vi "TestM1M3SALEvents.vi"() -> ()   [LabVIEW 2016]
uses:
  Communicator/M1M3SAL/M1M3SAL.lvclass
  Communicator/DataTypes/M1M3SALSettings.ctl
  UserEvents/UserEvents.lvclass
  DataTypes/General/ShutdownEvent.ctl
  Communicator/M1M3SAL/M1M3SAL.lvclass/M1M3SAL.ctl
  UserEvents/UserEvents.lvclass/UserEvents.ctl
  DataTypes/Topics/EventActuatorBroadcastCounter.ctl
  DataTypes/Topics/Parts/Timestamp.ctl
  DataTypes/Topics/EventActuatorTestStatus.ctl
  DataTypes/Topics/EventAirStatus.ctl
  DataTypes/Topics/EventAppliedSettingsMatchStart.ctl
  DataTypes/Topics/EventCellChecks.ctl
  DataTypes/Topics/EventDetailedState.ctl
  DataTypes/Topics/Parts/DetailedStates.ctl
  DataTypes/Topics/EventElevationAngleChecks.ctl
  DataTypes/Topics/EventForceActuatorSafetyChecks.ctl
  DataTypes/Topics/EventErrorCode.ctl
  DataTypes/Topics/EventForceActuatorInfo.ctl
  DataTypes/Topics/EventHardpointActuatorInfo.ctl
  DataTypes/Topics/EventForceActuatorTest.ctl
  DataTypes/Topics/Parts/TestStatus.ctl
  DataTypes/Topics/EventHardpointActuatorBreakaway.ctl
  DataTypes/Topics/EventHardpointActuatorChase.ctl
  DataTypes/Topics/EventILCCommunication.ctl
  DataTypes/Topics/EventLowerMirrorComplete.ctl
  DataTypes/Topics/EventRaiseMirrorComplete.ctl
  DataTypes/Topics/EventServoLoops.ctl
  DataTypes/Topics/EventSettingsApplied.ctl
  DataTypes/Topics/EventSettingVersions.ctl
  DataTypes/Topics/EventStartupChecks.ctl
  DataTypes/Topics/EventStatusChecks.ctl
  DataTypes/Topics/EventSummaryState.ctl
  DataTypes/Topics/Parts/SummaryStates.ctl
  Communicator/M1M3SupportCommunicator.lvlib
  DataTypes/Topics/M1M3SupportTopics.lvlib
  DataTypes/General/M1M3SupportGeneral.lvlib
panel:
  out "SummaryState":bool
  out "StatusChecks":bool
  out "StartupChecks":bool
  out "SettingVersions":bool
  out "SettingsApplied":bool
  out "ServoLoops":bool
  out "RaiseMirrorComplete":bool
  out "LowerMirrorComplete":bool
  out "ILCCommunication":bool
  out "HardpointActuatorInfo":bool
  out "HardpointActuatorChase":bool
  out "HardpointActuatorBreakaway":bool
  out "ForceActuatorTest":bool
  in  "SummaryStateGo":bool
  in  "StatusChecksGo":bool
  in  "StartupChecksGo":bool
  in  "SettingVersionsGo":bool
  in  "SettingsAppliedGo":bool
  in  "ServoLoopsGo":bool
  in  "RaiseMirrorCompleteGo":bool
  in  "LowerMirrorCompleteGo":bool
  in  "ILCCommunicationGo":bool
  in  "HardpointActuatorInfoGo":bool
  in  "HardpointActuatorChaseGo":bool
  in  "HardpointActuatorBreakawayGo":bool
  in  "ForceActuatorTestGo":bool
  out "ForceActuatorSafetyChecks":bool
  in  "ForceActuatorSafetyChecksGo":bool
  out "ForceActuatorInfo":bool
  out "ErrorCode":bool
  out "ElevationAngleChecks":bool
  in  "ForceActuatorInfoGo":bool
  in  "ErrorCodeGo":bool
  in  "ElevationAngleChecksGo":bool
  out "DetailedState":bool
  out "CellChecks":bool
  out "AppliedSettingsMatchStart":bool
  out "AirStatus":bool
  in  "DetailedStateGo":bool
  in  "CellChecksGo":bool
  in  "AppliedSettingsMatchStartGo":bool
  in  "AirStatusGo":bool
  in  "ActuatorTestStatusGo":bool
  out "ActuatorTestStatus":bool
  out "Ready?":bool
  in  "ActuatorBroadcastCounterGo":bool
  out "ActuatorBroadcastCounter":bool
  in  "Stop":bool
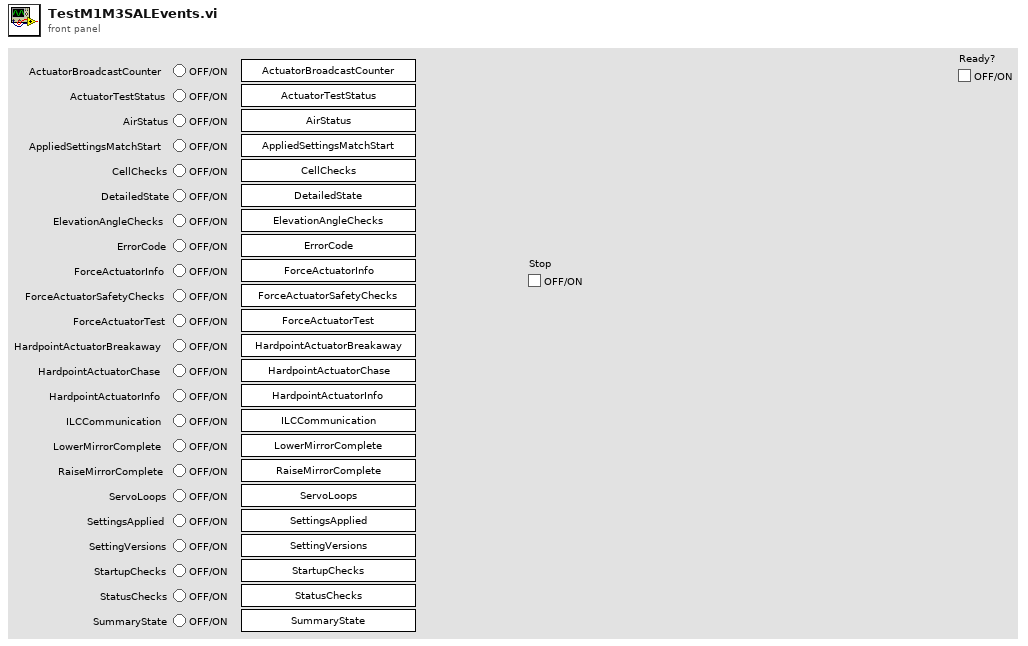
[diagram p1: front panel]
types:
  T1 = typedef "M1M3SupportGeneral.lvlib/ShutdownEvent.ctl" = cluster{"Shutdown":bool}
  T2 = typedef "M1M3SupportCommunicator.lvlib/M1M3SALSettings.ctl" = cluster{"IPAddress":string, "Port":u16, "StartupScript":string}
  T3 = typedef "M1M3SupportTopics.lvlib/Timestamp.ctl" = dbl
  T4 = typedef "M1M3SupportTopics.lvlib/DetailedStates.ctl" = enum16{"OfflineState", "InitialState", "StandbyState", "DisabledState", "ParkedState", "FaultState", "ParkedMaintenanceState", "ActiveMaintenanceState"}
  T5 = typedef "M1M3SupportTopics.lvlib/TestStatus.ctl" = enum16{"NotRun", "Pass", "Fail"}
  T6 = typedef "M1M3SupportTopics.lvlib/SummaryStates.ctl" = enum16{"OfflineState", "StandbyState", "DisabledState", "EnabledState", "FaultState"}
  T7 = typedef "M1M3SupportTypes.lvlib/Timestamp.ctl" = dbl
  T8 = typedef "M1M3SupportTypes.lvlib/SummaryStates.ctl" = enum16{"OfflineState", "StandbyState", "DisabledState", "EnabledState", "FaultState"}
  T9 = typedef "M1M3SupportTopics.lvlib/EventActuatorBroadcastCounter.ctl" = cluster{"Timestamp":T3, "ActuatorId":i32, "CounterOk":bool}
  T10 = typedef "M1M3SupportTopics.lvlib/EventActuatorTestStatus.ctl" = cluster{"Timestamp":T3, "AllTestsRan":bool}
  T11 = typedef "M1M3SupportTopics.lvlib/EventAirStatus.ctl" = cluster{"Timestamp":T3, "AirCommandedOn":bool, "AirOn":bool, "AirPressureOk":bool, "HardpointAirPressureOk":bool}
  T12 = typedef "M1M3SupportTopics.lvlib/EventAppliedSettingsMatchStart.ctl" = cluster{"Timestamp":T3, "AppliedSettingsMatchStart":bool}
  T13 = typedef "M1M3SupportTopics.lvlib/EventCellChecks.ctl" = cluster{"Timestamp":T3, "MirrorDoorClosed":bool}
  T14 = typedef "M1M3SupportTopics.lvlib/EventDetailedState.ctl" = cluster{"Timestamp":T3, "DetailedStates":T4}
  T15 = typedef "M1M3SupportTopics.lvlib/EventElevationAngleChecks.ctl" = cluster{"Timestamp":T3, "MatchesTMA":bool, "MatchesInclinometer":bool, "MatchesMeasured":bool}
  T16 = typedef "M1M3SupportTopics.lvlib/EventForceActuatorSafetyChecks.ctl" = cluster{"Timestamp":T3, "AllInSafetyLimit":bool, "SafetyLimitOk":bool[], "MirrorWeightOk":bool, "XMomentOk":bool, "YMomentOk":bool, "AllNeighborsOk":bool, "NeighborsOk":bool[], "MagnitudeOk":bool, "AllGlobalBendingOk":bool, "GlobalBendingOk":bool[], "FollowingErrorOk":bool, "AxialFollowingErrorOk":bool[], "LateralFollowingErrorOk":bool[], "AOSNetForceOk":bool, "AllElevationForcesOk":bool, "ElevationForcesOk":bool[], "AllAzimuthForcesOk":bool, "AzimuthForcesOk":bool[], "AllThermalForcesOk":bool, "ThermalForcesOk":bool[], "AllAOSForcesOk":bool, "AOSForcesOk":bool[]}
  T17 = typedef "M1M3SupportTopics.lvlib/EventErrorCode.ctl" = cluster{"Timestamp":T3, "ErrorCode":i32}
  T18 = typedef "M1M3SupportTopics.lvlib/EventForceActuatorInfo.ctl" = cluster{"Timestamp":T3, "ReferenceId":i32[], "XPosition":sgl[], "YPosition":sgl[], "ZPosition":sgl[], "ILCUniqueId":i64[], "ILCApplicationType":u8[], "NetworkNodeType":u8[], "ILCSelectedOptions":u8[], "NetworkNodeOptions":u8[], "MajorRevision":u8[], "MinorRevision":u8[], "ADCScanRate":u8[], "MainADCCalibrationK1":sgl[], "MainADCCalibrationK2":sgl[], "MainADCCalibrationK3":sgl[], "MainADCCalibrationK4":sgl[], "MainAxialLoadCellOffset":sgl[], "MainLateralLoadCellOffset":sgl[], "MainAxialLoadCellSensitivity":sgl[], "MainLateralLoadCellSensitivity":sgl[], "BackupADCCalibrationK1":sgl[], "BackupADCCalibrationK2":sgl[], "BackupADCCalibrationK3":sgl[], "BackupADCCalibrationK4":sgl[], "BackupAxialLoadCellOffset":sgl[], "BackupLateralLoadCellOffset":sgl[], "BackupAxialLoadCellSensitivity":sgl[], "BackupLateralLoadCellSensitivity":sgl[], "DCAAxialGain":sgl[], "DCALateralGain":sgl[], "DCAUniqueId":i64[], "DCAFirmwareType":u8[], "DCAMajorRevision":u8[], "DCAMinorRevision":u8[], "MainCalibrationError":bool[], "BackupCalibrationError":bool[], "DCAFirmwareUpdate":bool[], "UniqueIdCRCError":bool[], "ApplicationTypeMismatch":bool[], "ApplicationMissing":bool[], "ApplicationCRCMismatch":bool[], "OneWireMissing":bool[], "OneWire1Mismatch":bool[], "OneWire2Mismatch":bool[], "DCAUniqueIdCRCError":bool[], "DCAMainCalibrationError":bool[], "DCABackupCalibrationError":bool[], "DCAApplicationMissing":bool[], "DCAApplicationCRCMismatch":bool[], "DCABootloaderActive":bool[]}
  T19 = typedef "M1M3SupportTopics.lvlib/EventHardpointActuatorInfo.ctl" = cluster{"Timestamp":T3, "ReferenceId":i32[], "ReferencePosition":i32[], "XPosition":sgl[], "YPosition":sgl[], "ZPosition":sgl[], "ILCUniqueId":i64[], "ILCApplicationType":u8[], "NetworkNodeType":u8[], "ILCSelectedOptions":u8[], "NetworkNodeOptions":u8[], "MajorRevision":u8[], "MinorRevision":u8[], "ADCScanRate":u8[], "MainADCCalibrationK1":sgl[], "MainADCCalibrationK2":sgl[], "MainADCCalibrationK3":sgl[], "MainADCCalibrationK4":sgl[], "MainLoadCellOffset":sgl[], "MainLoadCellSensitivity":sgl[], "BackupADCCalibrationK1":sgl[], "BackupADCCalibrationK2":sgl[], "BackupADCCalibrationK3":sgl[], "BackupADCCalibrationK4":sgl[], "BackupLoadCellOffset":sgl[], "BackupLoadCellSensitivity":sgl[], "MainCalibrationError":bool[], "BackupCalibrationError":bool[], "UniqueIdCRCError":bool[], "ApplicationTypeMismatch":bool[], "ApplicationMissing":bool[], "ApplicationCRCMismatch":bool[], "OneWireMissing":bool[], "OneWire1Mismatch":bool[], "OneWire2Mismatch":bool[]}
  T20 = typedef "M1M3SupportTopics.lvlib/EventForceActuatorTest.ctl" = cluster{"Timestamp":T3, "ActuatorId":i32, "TestStatus":T5}
  T21 = typedef "M1M3SupportTopics.lvlib/EventHardpointActuatorBreakaway.ctl" = cluster{"Timestamp":T3, "ActuatorId":i32, "ForceOk":bool}
  T22 = typedef "M1M3SupportTopics.lvlib/EventHardpointActuatorChase.ctl" = cluster{"Timestamp":T3, "ActuatorId":i32, "Chasing":bool}
  T23 = typedef "M1M3SupportTopics.lvlib/EventILCCommunication.ctl" = cluster{"Timestamp":T3, "ActuatorId":i32, "CommunicationOK":bool}
  T24 = typedef "M1M3SupportTopics.lvlib/EventLowerMirrorComplete.ctl" = cluster{"Timestamp":T3, "Successful":bool}
  T25 = typedef "M1M3SupportTopics.lvlib/EventRaiseMirrorComplete.ctl" = cluster{"Timestamp":T3, "Successful":bool}
  T26 = typedef "M1M3SupportTopics.lvlib/EventServoLoops.ctl" = cluster{"Timestamp":T3, "HardpointChase":bool, "HardpointOffloading":bool, "OuterLoopTimeOk":bool}
  T27 = typedef "M1M3SupportTopics.lvlib/EventSettingsApplied.ctl" = cluster{"Timestamp":T3, "Settings":string}
  T28 = typedef "M1M3SupportTopics.lvlib/EventSettingVersions.ctl" = cluster{"Timestamp":T3, "RecommendedSettingsVersion":string}
  T29 = typedef "M1M3SupportTopics.lvlib/EventStartupChecks.ctl" = cluster{"Timestamp":T3, "ILCVersionsOk":bool, "DCAVersionsOk":bool, "ILCFirmwareOk":bool, "DCAFirmwareOk":bool, "ILCStatusOk":bool, "DCAStatusOk":bool}
  T30 = typedef "M1M3SupportTopics.lvlib/EventStatusChecks.ctl" = cluster{"Timestamp":T3, "ILCResetOk":bool, "DCAResetOk":bool, "ILCPowerOk":bool, "DCAPowerOk":bool}
  T31 = typedef "M1M3SupportTopics.lvlib/EventSummaryState.ctl" = cluster{"Timestamp":T3, "SummaryStates":T6}
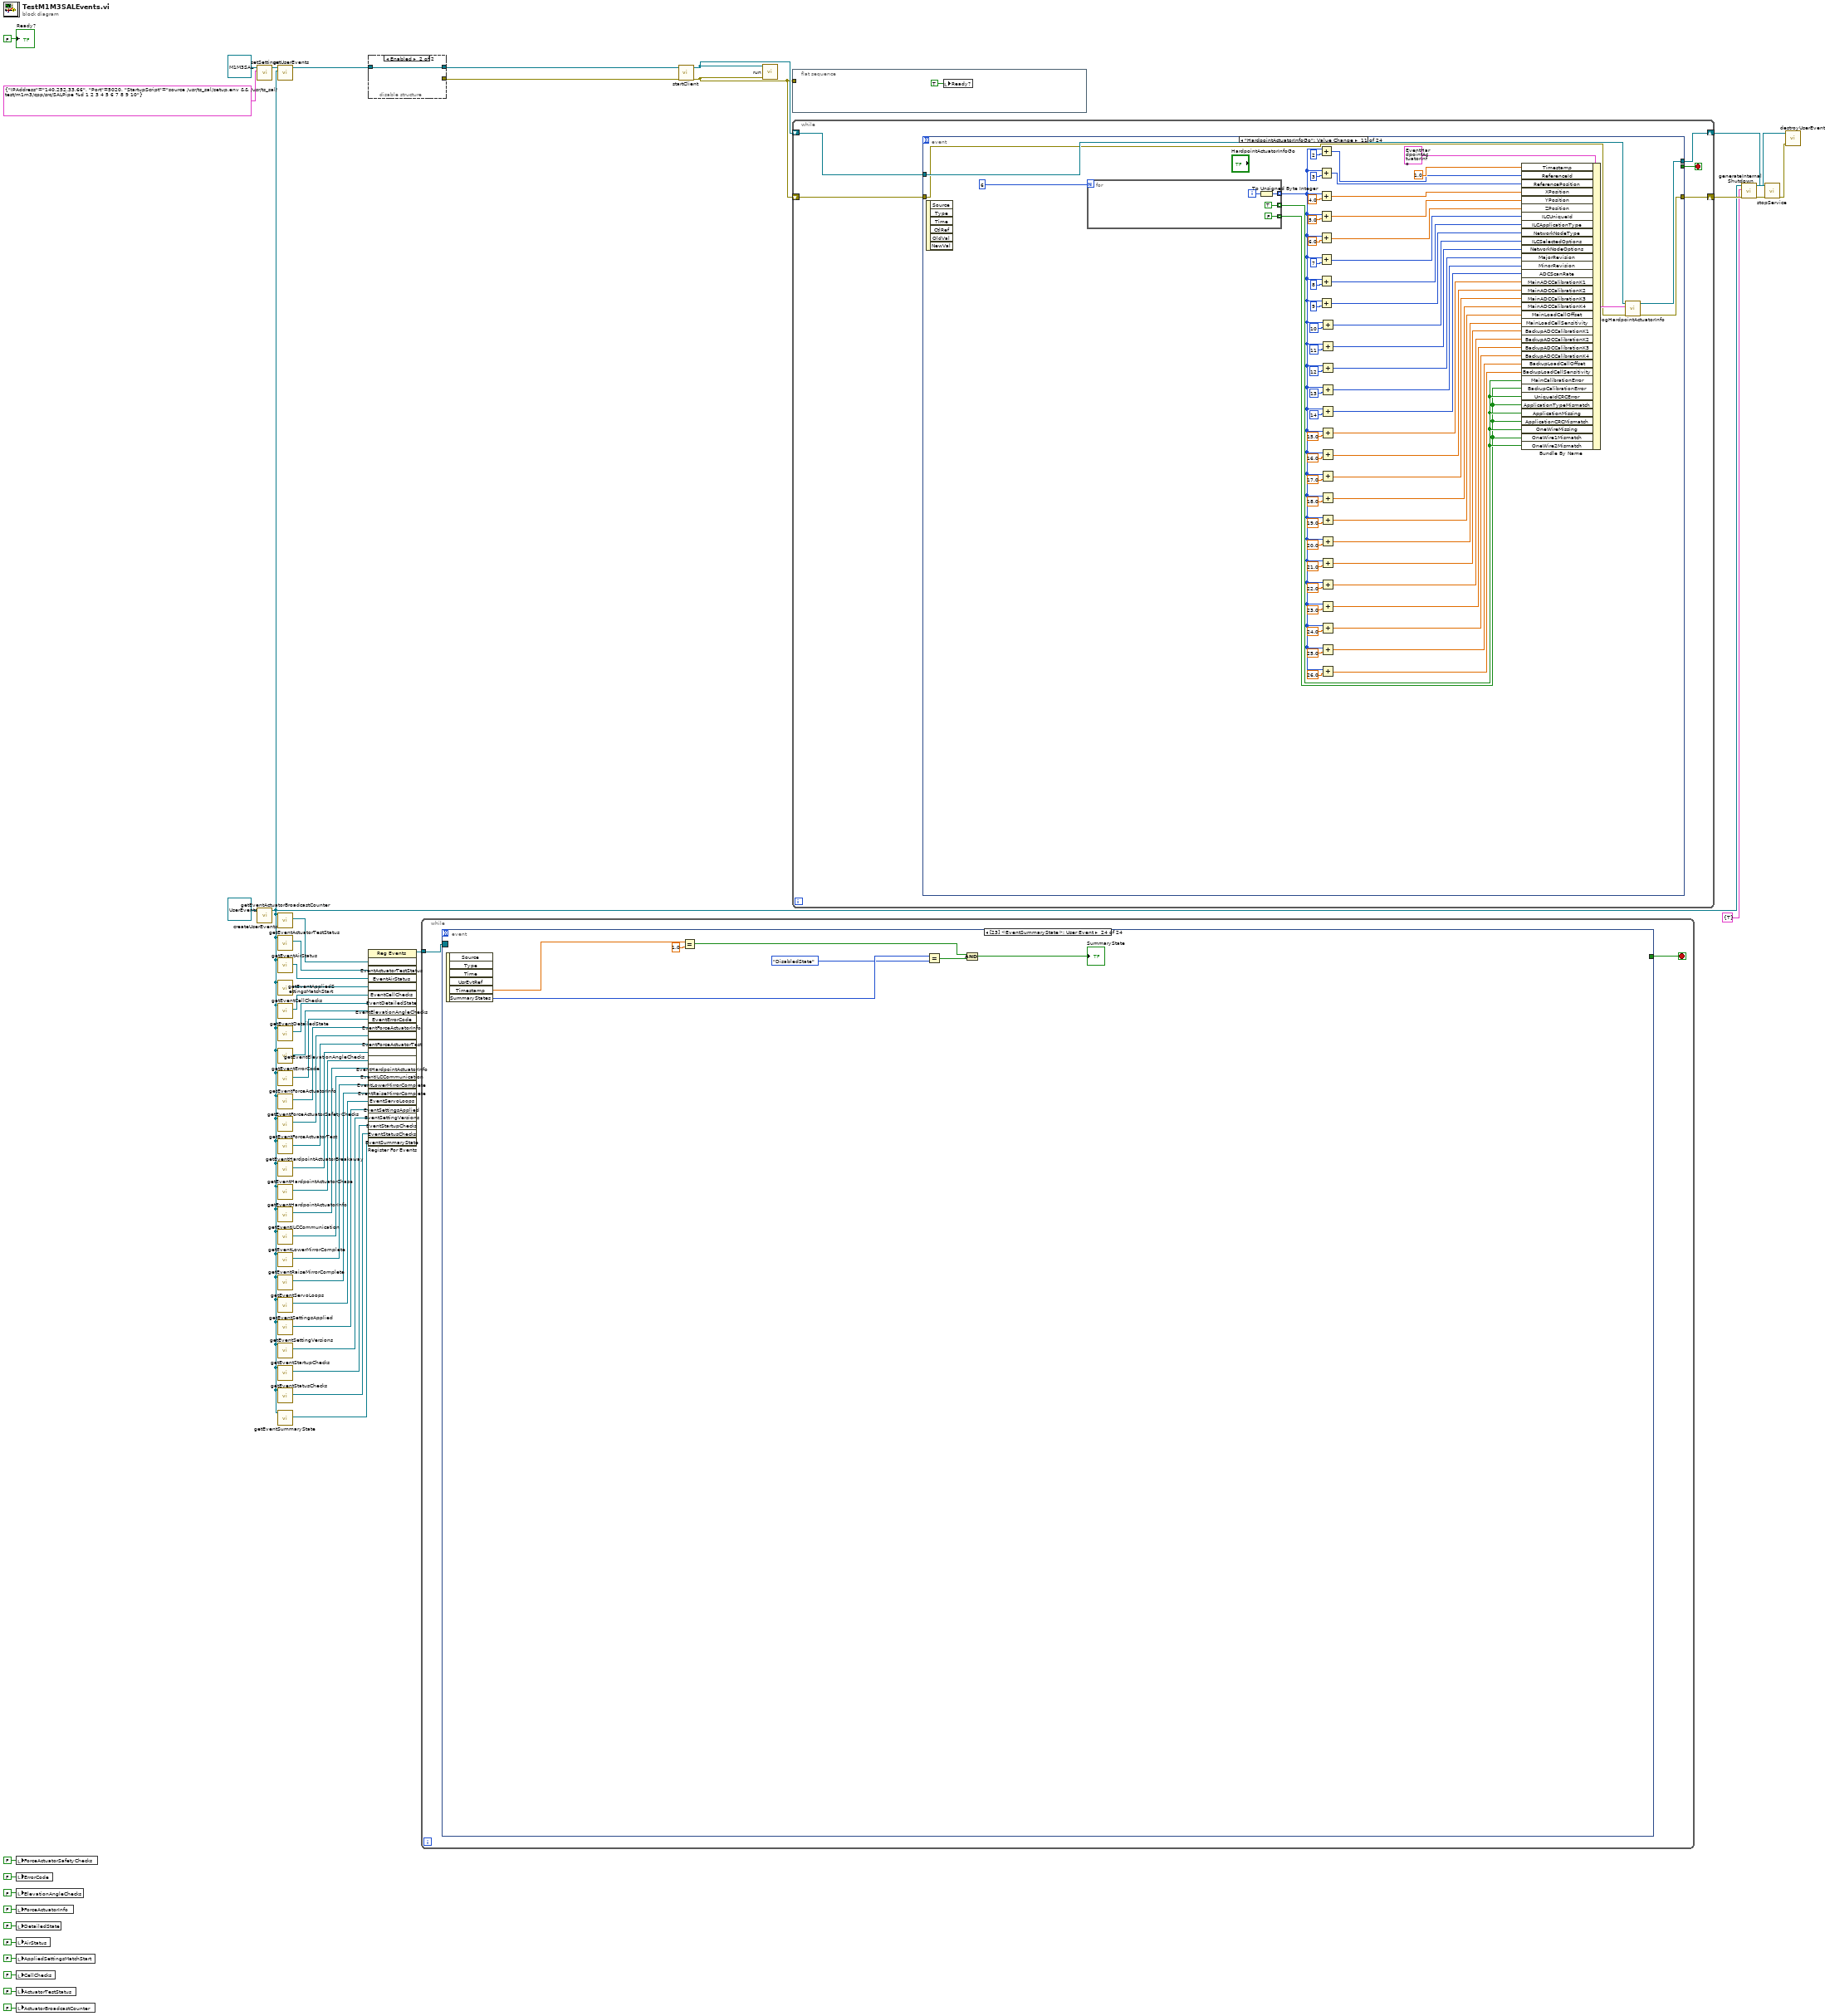
[diagram p0: block diagram]
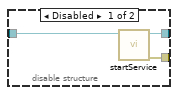
[diagram p2: hidden frame]
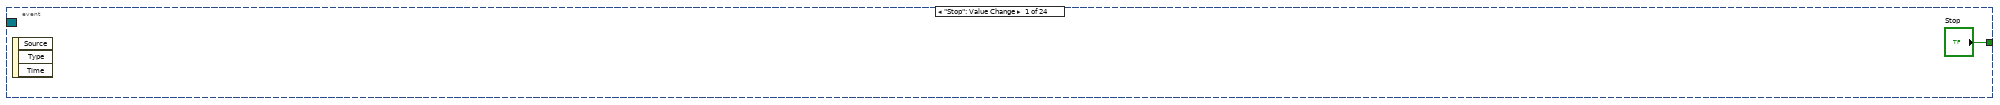
[diagram p3: hidden frame]
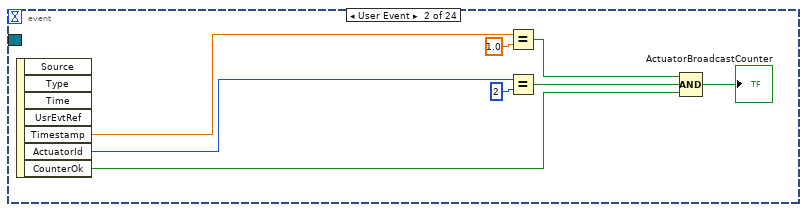
[diagram p4: hidden frame]
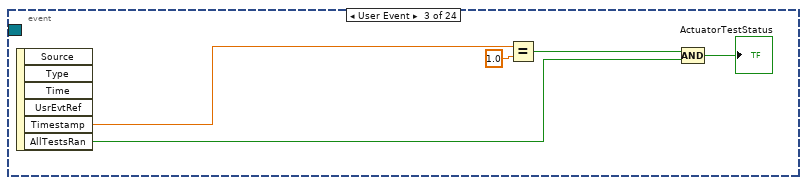
[diagram p5: hidden frame]
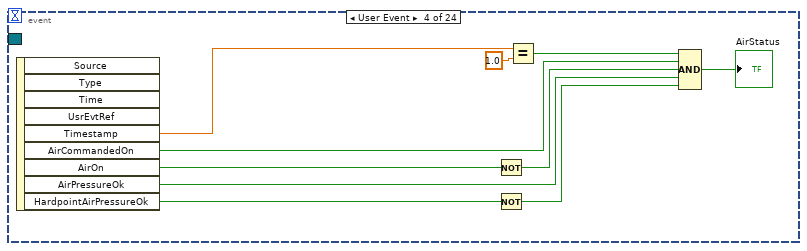
[diagram p6: hidden frame]
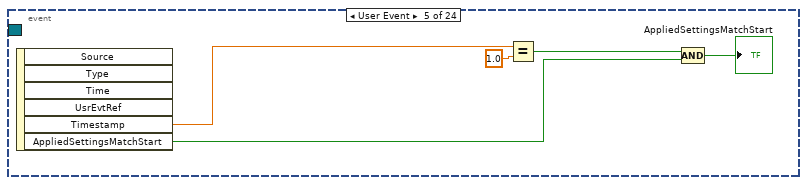
[diagram p7: hidden frame]
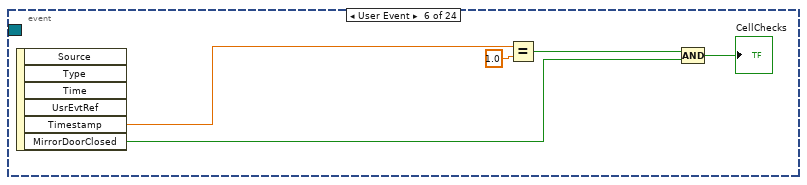
[diagram p8: hidden frame]
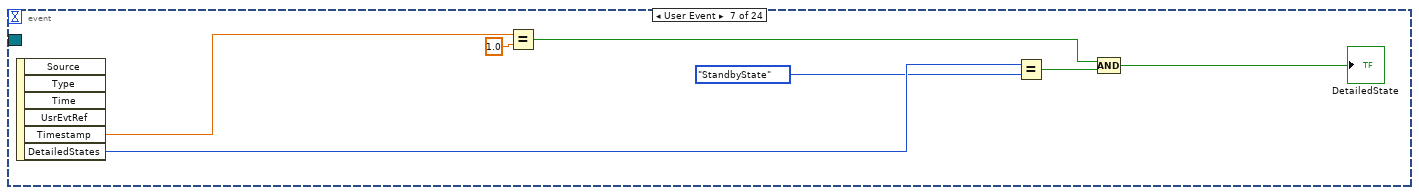
[diagram p9: hidden frame]
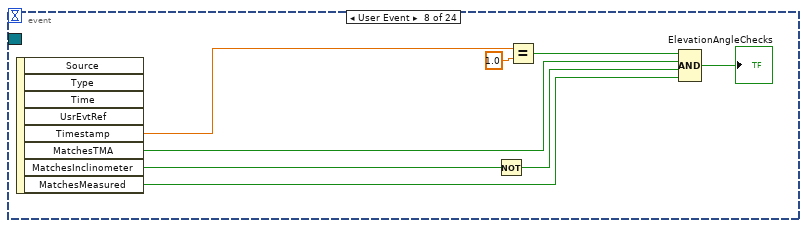
[diagram p10: hidden frame]
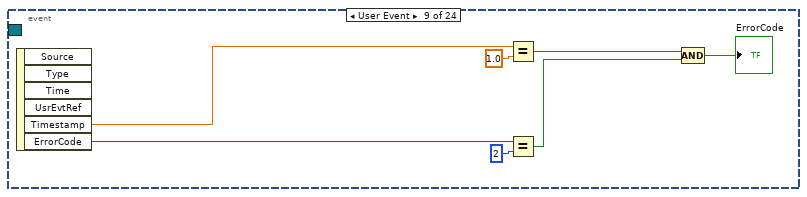
[diagram p11: hidden frame]
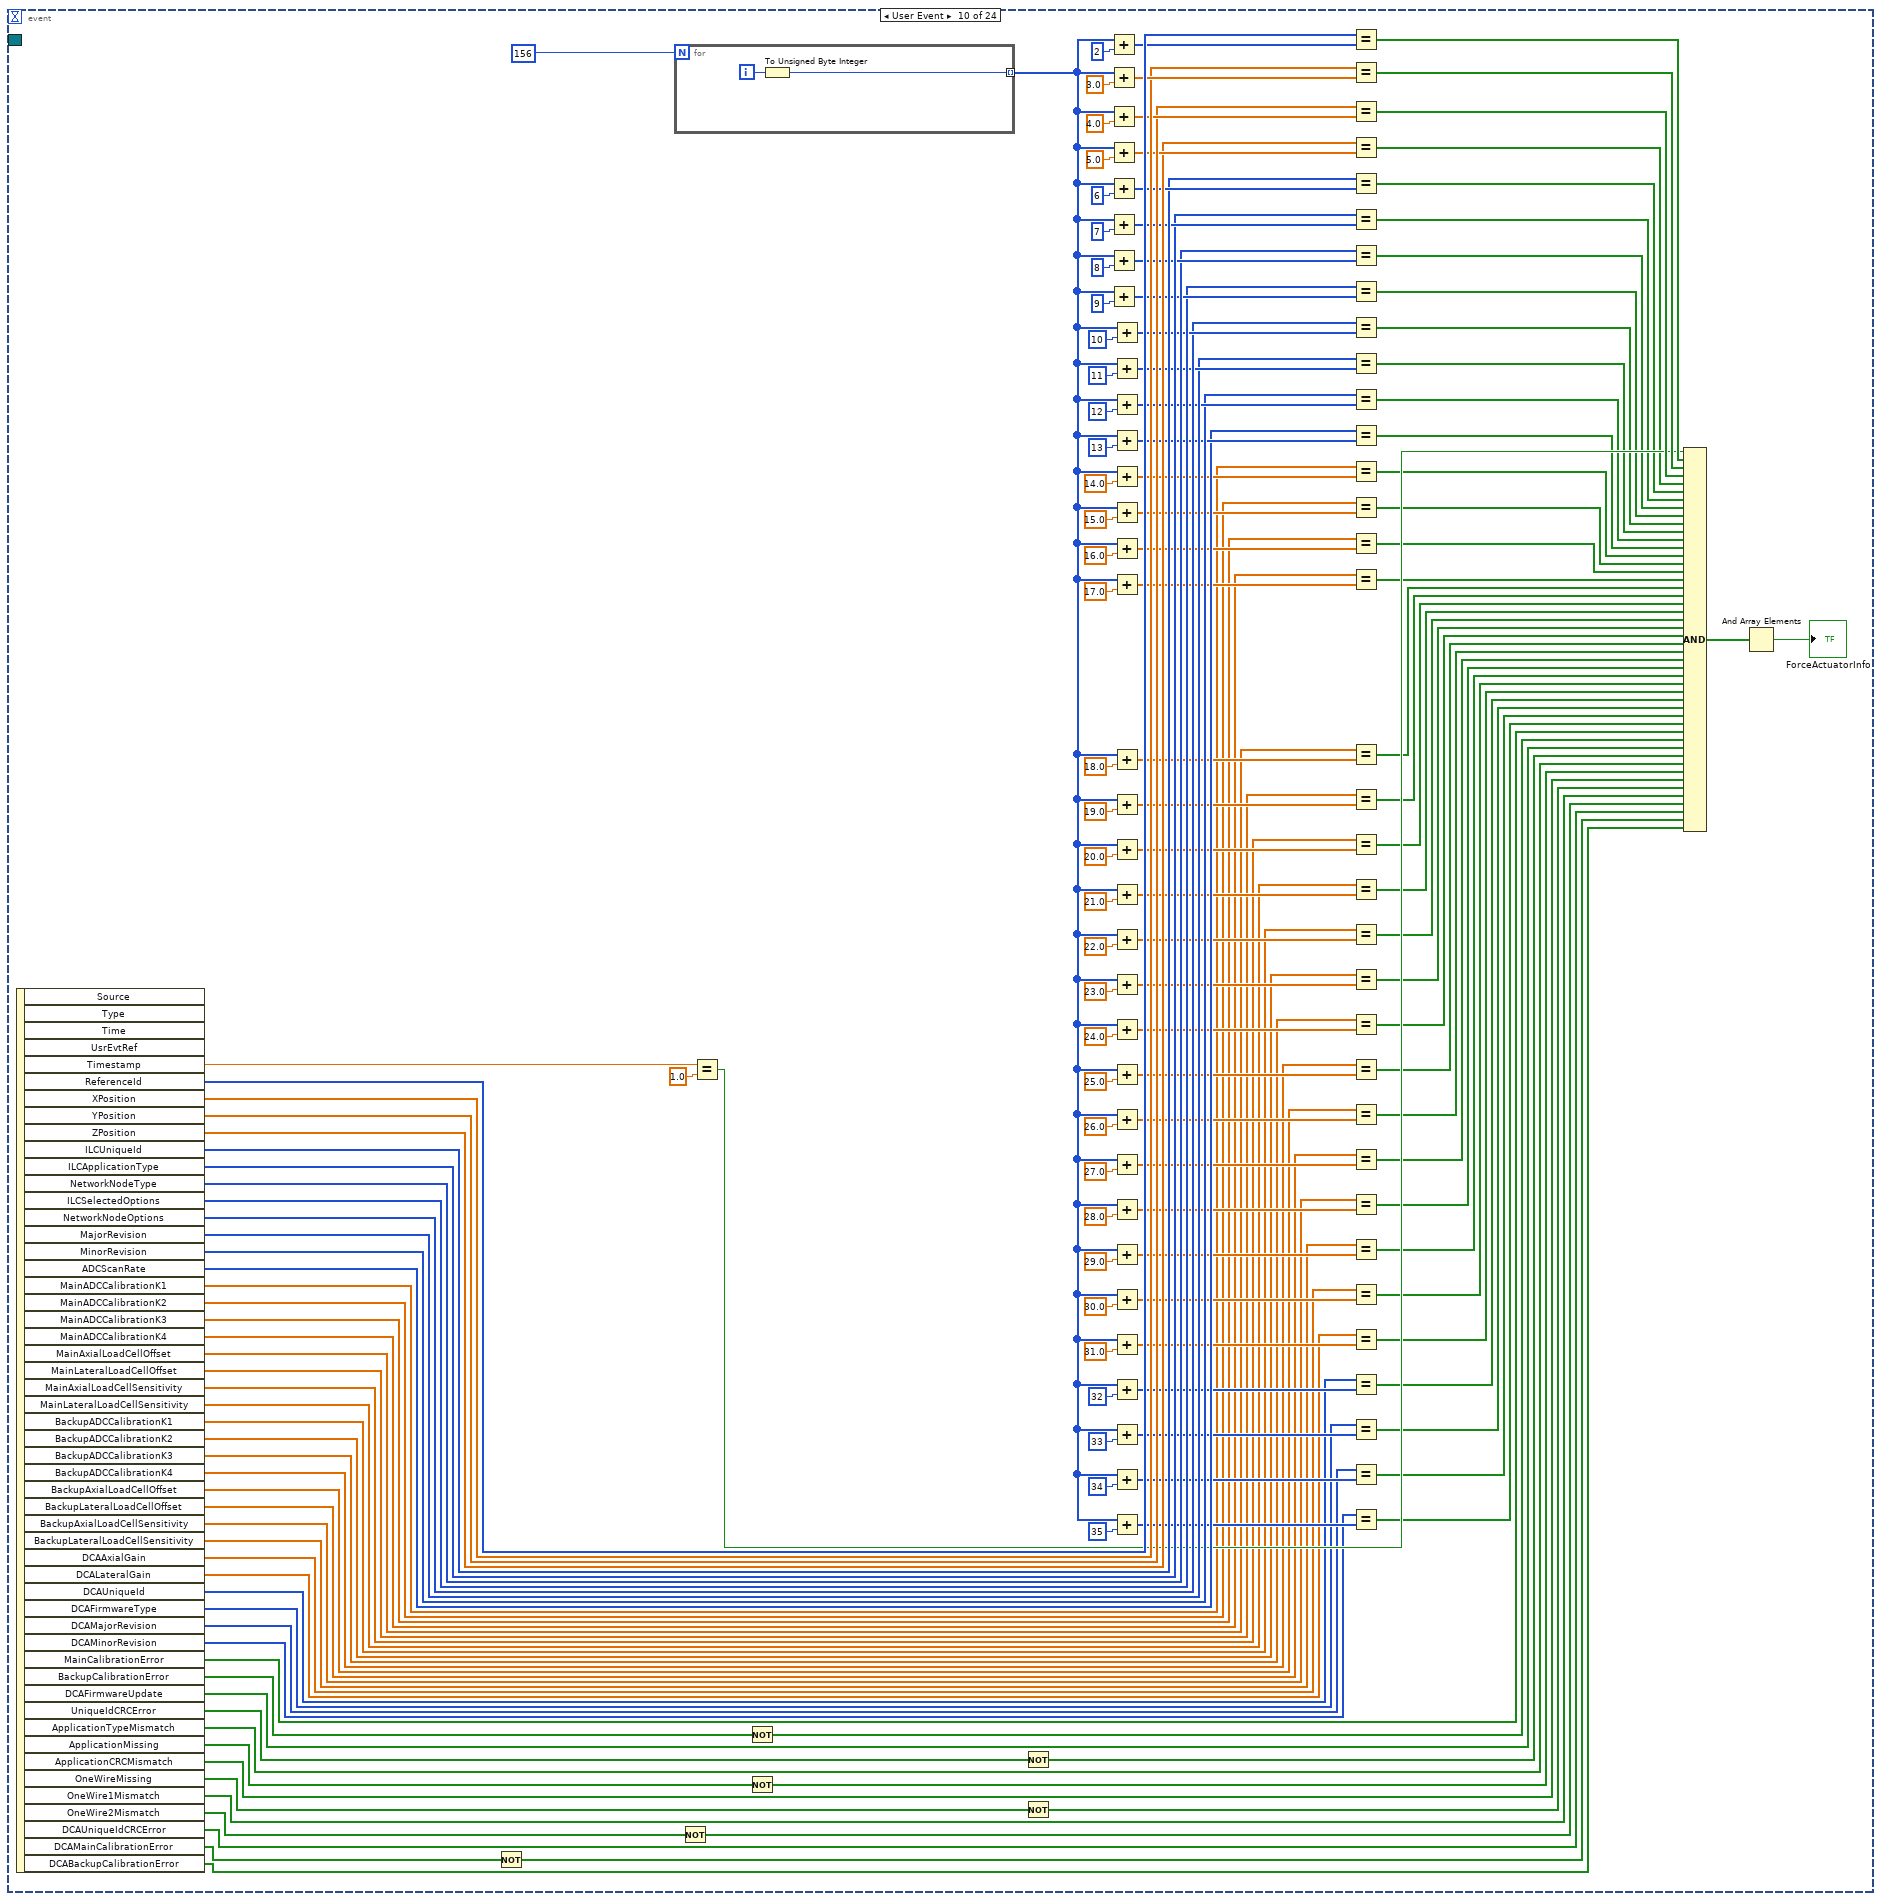
[diagram p12: hidden frame]
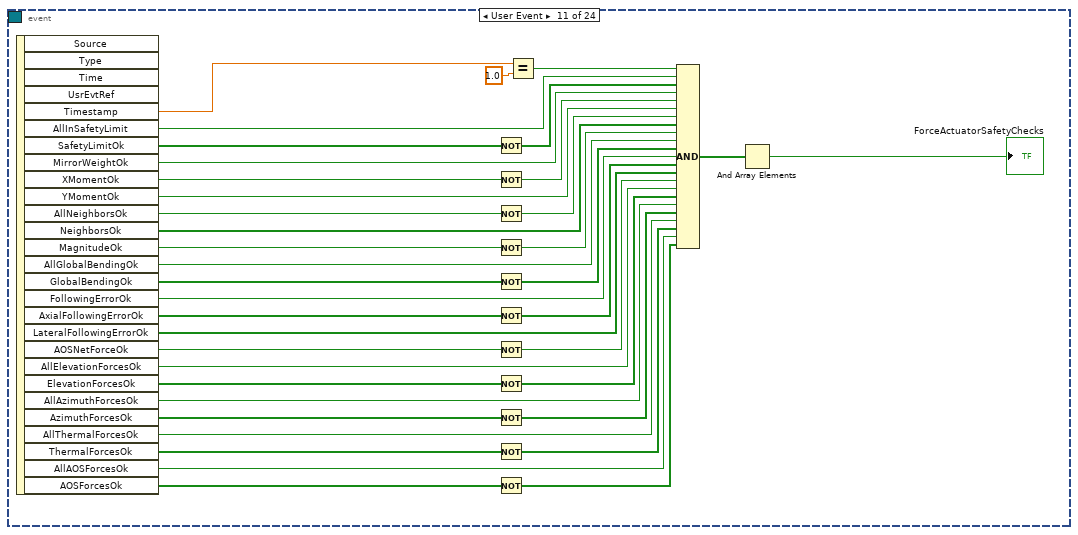
[diagram p13: hidden frame]
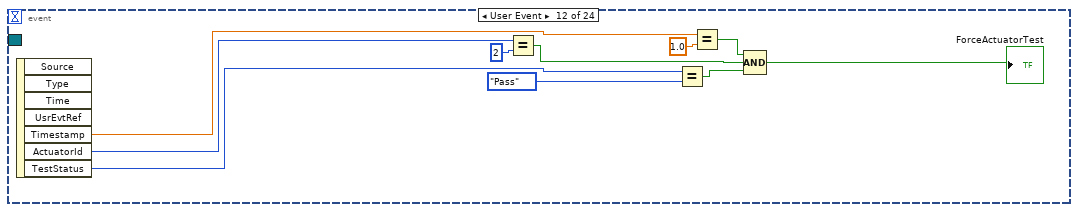
[diagram p14: hidden frame]
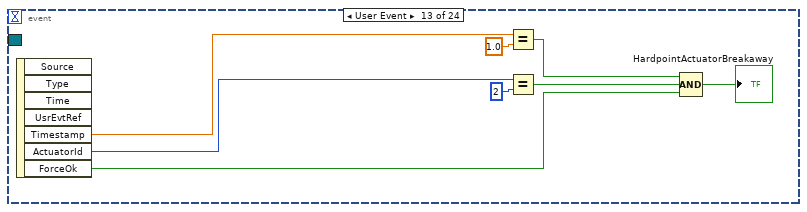
[diagram p15: hidden frame]
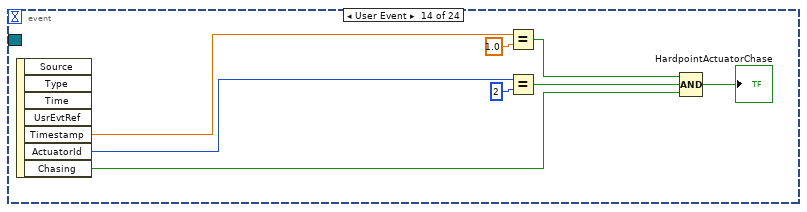
[diagram p16: hidden frame]
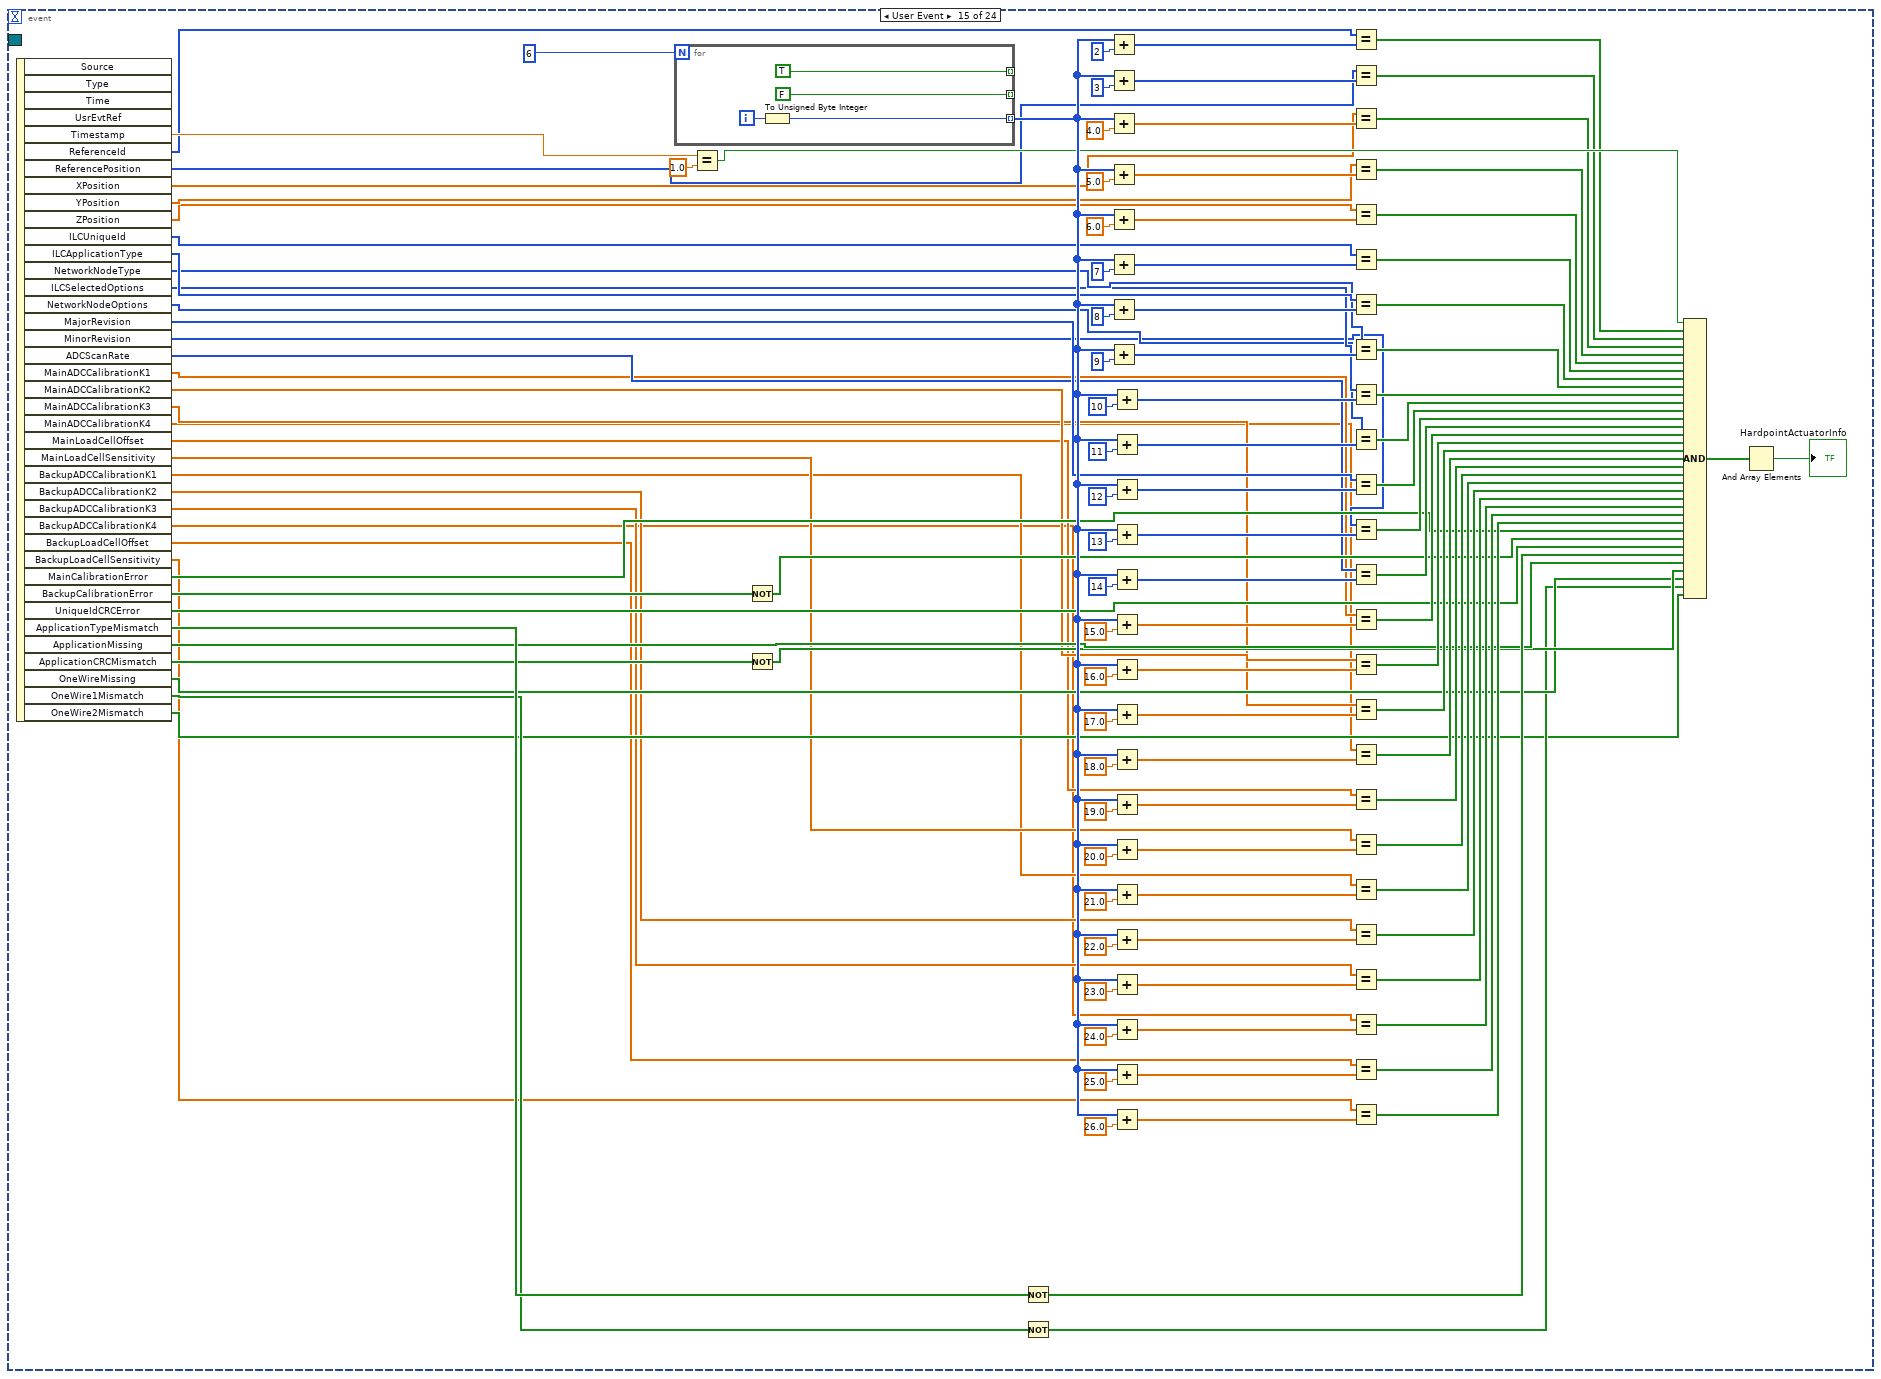
[diagram p17: hidden frame]
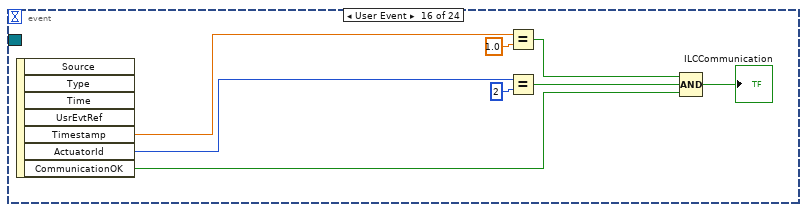
[diagram p18: hidden frame]
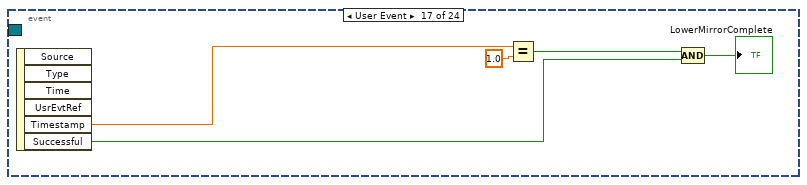
[diagram p19: hidden frame]
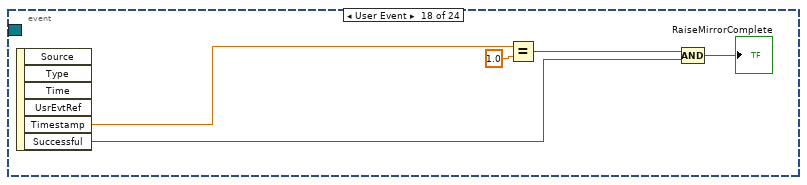
[diagram p20: hidden frame]
diagram:
  n1 = local write "ForceActuatorSafetyChecks"(FALSE ("TelemetryMirrorForceData")) -> ()
  n2 = local write "ErrorCode"(FALSE ("TelemetryHardpointData")) -> ()
  n3 = local write "ElevationAngleChecks"(FALSE ("TelemetryFPGAData")) -> ()
  n4 = local write "ForceActuatorInfo"(FALSE ("TelemetryHardpointStatus")) -> ()
  n5 = local write "DetailedState"(FALSE ("TelemetryForceActuatorStatus")) -> ()
  n6 = local write "AirStatus"(FALSE ("TelemetryDynamicData")) -> ()
  n7 = local write "AppliedSettingsMatchStart"(FALSE ("TelemetryElevationData")) -> ()
  n8 = local write "CellChecks"(FALSE ("TelemetryForceActuatorData")) -> ()
  n9 = local write "ActuatorTestStatus"(FALSE ("TelemetryIMSData")) -> ()
  n10 = local write "ActuatorBroadcastCounter"(FALSE ("TelemetryAirData")) -> ()
  n11 = call "setSettings.vi"("Settings"=T2 {"IPAddress"="140.252.33.66", "Port"=5020, "StartupScript"="source /usr/ts_sal/setup.env && /usr/ts_sal/test/m1m3/cpp/src/SALPipe %d 1 2 3 4 5 6 7 8 9 10"}, "M1M3SAL in"=refnum<class "M1M3SAL.lvclass"> refnum ("M1M3SupportCommunicator.lvlib:M1M3SAL.lvclass")) -> ("M1M3SAL out"=w48:refnum<class "M1M3SAL.lvclass">)  [unwired: 9 in]
  n12 = call "createUserEvents.vi"("UserEvents in"=refnum<class "UserEvents.lvclass"> refnum ("UserEvents.lvclass")) -> ("UserEvents out"=w24:refnum<class "UserEvents.lvclass">)  [unwired: 9 in, 1 out]
  n13 = call "setUserEvents.vi"("UserEvents"=w24, "M1M3SAL in"=w48) -> ("M1M3SAL out"=w47:refnum<class "M1M3SAL.lvclass">)  [unwired: 9 in]
  n14 = call "getEventActuatorBroadcastCounter.vi"("UserEvents in"=w24) -> ("EventActuatorBroadcastCounter"=w23:refnum<user-event>)  [unwired: 9 in, 1 out]
  n15 = call "getEventActuatorTestStatus.vi"("UserEvents in"=w24) -> ("EventActuatorTestStatus"=w22:refnum<user-event>)  [unwired: 9 in, 1 out]
  n16 = call "getEventAirStatus.vi"("UserEvents in"=w24) -> ("EventAirStatus"=w21:refnum<user-event>)  [unwired: 9 in, 1 out]
  n17 = call "getEventAppliedSettingsMatchStart.vi"("UserEvents in"=w24) -> ("EventAppliedSettingsMatchStart"=w20:refnum<user-event>)  [unwired: 9 in, 1 out]
  n18 = call "getEventCellChecks.vi"("UserEvents in"=w24) -> ("EventCellChecks"=w19:refnum<user-event>)  [unwired: 9 in, 1 out]
  n19 = call "getEventDetailedState.vi"("UserEvents in"=w24) -> ("EventDetailedState"=w18:refnum<user-event>)  [unwired: 9 in, 1 out]
  n20 = call "getEventElevationAngleChecks.vi"("UserEvents in"=w24) -> ("EventElevationAngleChecks"=w17:refnum<user-event>)  [unwired: 9 in, 1 out]
  n21 = call "getEventErrorCode.vi"("UserEvents in"=w24) -> ("EventErrorCode"=w16:refnum<user-event>)  [unwired: 9 in, 1 out]
  n22 = call "getEventForceActuatorInfo.vi"("UserEvents in"=w24) -> ("EventForceActuatorInfo"=w15:refnum<user-event>)  [unwired: 9 in, 1 out]
  n23 = call "getEventForceActuatorSafetyChecks.vi"("UserEvents in"=w24) -> ("EventForceActuatorSafetyChecks"=w14:refnum<user-event>)  [unwired: 9 in, 1 out]
  n24 = call "getEventForceActuatorTest.vi"("UserEvents in"=w24) -> ("EventForceActuatorTest"=w13:refnum<user-event>)  [unwired: 9 in, 1 out]
  n25 = call "getEventHardpointActuatorBreakaway.vi"("UserEvents in"=w24) -> ("EventHardpointActuatorBreakaway"=w12:refnum<user-event>)  [unwired: 9 in, 1 out]
  n26 = call "getEventHardpointActuatorChase.vi"("UserEvents in"=w24) -> ("EventHardpointActuatorChase"=w11:refnum<user-event>)  [unwired: 9 in, 1 out]
  n27 = call "getEventHardpointActuatorInfo.vi"("UserEvents in"=w24) -> ("EventHardpointActuatorInfo"=w10:refnum<user-event>)  [unwired: 9 in, 1 out]
  n28 = call "getEventILCCommunication.vi"("UserEvents in"=w24) -> ("EventILCCommunication"=w9:refnum<user-event>)  [unwired: 9 in, 1 out]
  n29 = call "getEventLowerMirrorComplete.vi"("UserEvents in"=w24) -> ("EventLowerMirrorComplete"=w8:refnum<user-event>)  [unwired: 9 in, 1 out]
  n30 = call "getEventRaiseMirrorComplete.vi"("UserEvents in"=w24) -> ("EventRaiseMirrorComplete"=w7:refnum<user-event>)  [unwired: 9 in, 1 out]
  n31 = call "getEventServoLoops.vi"("UserEvents in"=w24) -> ("EventServoLoops"=w6:refnum<user-event>)  [unwired: 9 in, 1 out]
  n32 = call "getEventSettingsApplied.vi"("UserEvents in"=w24) -> ("EventSettingsApplied"=w5:refnum<user-event>)  [unwired: 9 in, 1 out]
  n33 = call "getEventSettingVersions.vi"("UserEvents in"=w24) -> ("EventSettingVersions"=w4:refnum<user-event>)  [unwired: 9 in, 1 out]
  n34 = call "getEventStartupChecks.vi"("UserEvents in"=w24) -> ("EventStartupChecks"=w3:refnum<user-event>)  [unwired: 9 in, 1 out]
  n35 = call "getEventStatusChecks.vi"("UserEvents in"=w24) -> ("EventStatusChecks"=w2:refnum<user-event>)  [unwired: 9 in, 1 out]
  n36 = call "getEventSummaryState.vi"("UserEvents in"=w24) -> ("EventSummaryState"=w1:refnum<user-event>)  [unwired: 9 in, 1 out]
  n37 = disable-structure shown="Enabled" {
    disable-tunnel: w47 -> [w54 w55]
    disable-tunnel: [w53 w55] -> w46
    disable-tunnel: [w52 _] -> w44
    frame Disabled {
      n38 = call-dynamic "startService.vi"("M1M3SAL in"=w54) -> ("error out"=w52:errorcluster, "M1M3SAL out"=w53:refnum<class "M1M3SAL.lvclass">)  [unwired: 9 in]
    }
    frame Enabled {
    }
  }
  n39 = register-events(w23, w22, w21, w20, w19, w18, w17, w16, w15, w14, w13, w12, w11, w10, w9, w8, w7, w6, w5, w4, w3, w2, w1) -> (reference out=w45:refnum<event-registration>)  [unwired: 2 in, 1 out]
  n40 = while {
    tunnel: w45 -> [w57]
    stop <- w56 stop-if-true
    n41 = event shown="[23] <EventSummaryState>: User Event" {
      selector: w57 -> [_ _ _ _ _ _ _ _ _ _ _ _ _ _ _ _ _ _ _ _ _ _ _ _]
      dyn-events: _ -> [_ _ _ _ _ _ _ _ _ _ _ _ _ _ _ _ _ _ _ _ _ _ _ _]
      timeout: _ -> [_ _ _ _ _ _ _ _ _ _ _ _ _ _ _ _ _ _ _ _ _ _ _ _]
      tunnel: ["Stop" _ _ _ _ _ _ _ _ _ _ _ _ _ _ _ _ _ _ _ _ _ _ _] -> w56
      event "Stop": Value Change {
        n42 = event-data() -> ()  [unwired: 1 in, 3 out]
      }
      event User Event {
        n43 = event-data() -> ("Timestamp"=w66:T3, "ActuatorId"=w64:i32, "CounterOk"=w60:bool)  [unwired: 1 in, 4 out]
        n44 = Equal?(x=w66, y=T3 1.0) -> (x = y?=w62:bool)
        n45 = Equal?(x=w64, y=2) -> (x = y?=w61:bool)
        n46 = Compound Arithmetic op=AND(w62, w61, w60) -> (→"ActuatorBroadcastCounter":bool)
      }
      event User Event {
        n47 = event-data() -> ("Timestamp"=w71:T3, "AllTestsRan"=w68:bool)  [unwired: 1 in, 4 out]
        n48 = Equal?(x=w71, y=T3 1.0) -> (x = y?=w69:bool)
        n49 = Compound Arithmetic op=AND(w69, w68) -> (→"ActuatorTestStatus":bool)
      }
      event User Event {
        n50 = event-data() -> ("Timestamp"=w81:T3, "AirCommandedOn"=w78:bool, "AirOn"=w77:bool, "AirPressureOk"=w75:bool, "HardpointAirPressureOk"=w74:bool)  [unwired: 1 in, 4 out]
        n51 = Not(x=w77) -> (.not. x?=w76:bool)
        n52 = Not(x=w74) -> (.not. x?=w73:bool)
        n53 = Equal?(x=w81, y=T3 1.0) -> (x = y?=w79:bool)
        n54 = Compound Arithmetic op=AND(w79, w78, w76, w75, w73) -> (→"AirStatus":bool)
      }
      event User Event {
        n55 = event-data() -> ("Timestamp"=w86:T3, "AppliedSettingsMatchStart"=w83:bool)  [unwired: 1 in, 4 out]
        n56 = Equal?(x=w86, y=T3 1.0) -> (x = y?=w84:bool)
        n57 = Compound Arithmetic op=AND(w84, w83) -> (→"AppliedSettingsMatchStart":bool)
      }
      event User Event {
        n58 = event-data() -> ("Timestamp"=w91:T3, "MirrorDoorClosed"=w89:bool)  [unwired: 1 in, 4 out]
        n59 = Equal?(x=w91, y=T3 1.0) -> (x = y?=w88:bool)
        n60 = Compound Arithmetic op=AND(w88, w89) -> (→"CellChecks":bool)
      }
      event User Event {
        n61 = event-data() -> ("Timestamp"=w98:T3, "DetailedStates"=w97:T4)  [unwired: 1 in, 4 out]
        n62 = Equal?(x=w98, y=T3 1.0) -> (x = y?=w94:bool)
        n63 = Equal?(x=w97, y=DetailedStates."StandbyState") -> (x = y?=w93:bool)
        n64 = Compound Arithmetic op=AND(w94, w93) -> (→"DetailedState":bool)
      }
      event User Event {
        n65 = event-data() -> ("Timestamp"=w106:T3, "MatchesTMA"=w103:bool, "MatchesInclinometer"=w102:bool, "MatchesMeasured"=w100:bool)  [unwired: 1 in, 4 out]
        n66 = Not(x=w102) -> (.not. x?=w101:bool)
        n67 = Equal?(x=w106, y=T3 1.0) -> (x = y?=w104:bool)
        n68 = Compound Arithmetic op=AND(w104, w103, w101, w100) -> (→"ElevationAngleChecks":bool)
      }
      event User Event {
        n69 = event-data() -> ("Timestamp"=w113:T3, "ErrorCode"=w111:i32)  [unwired: 1 in, 4 out]
        n70 = Equal?(x=w113, y=T3 1.0) -> (x = y?=w109:bool)
        n71 = Equal?(x=w111, y=2) -> (x = y?=w108:bool)
        n72 = Compound Arithmetic op=AND(w109, w108) -> (→"ErrorCode":bool)
      }
      event User Event {
        n73 = event-data() -> ("Timestamp"=w212:T3, "ReferenceId"=w239:i32[], "XPosition"=w236:sgl[], "YPosition"=w234:sgl[], "ZPosition"=w232:sgl[], "ILCUniqueId"=w230:i64[], "ILCApplicationType"=w228:u8[], "NetworkNodeType"=w226:u8[], "ILCSelectedOptions"=w224:u8[], "NetworkNodeOptions"=w222:u8[], "MajorRevision"=w220:u8[], "MinorRevision"=w218:u8[], "ADCScanRate"=w216:u8[], "MainADCCalibrationK1"=w137:sgl[], "MainADCCalibrationK2"=w136:sgl[], "MainADCCalibrationK3"=w135:sgl[], "MainADCCalibrationK4"=w134:sgl[], "MainAxialLoadCellOffset"=w133:sgl[], "MainLateralLoadCellOffset"=w132:sgl[], "MainAxialLoadCellSensitivity"=w131:sgl[], "MainLateralLoadCellSensitivity"=w130:sgl[], "BackupADCCalibrationK1"=w129:sgl[], "BackupADCCalibrationK2"=w128:sgl[], "BackupADCCalibrationK3"=w127:sgl[], "BackupADCCalibrationK4"=w126:sgl[], "BackupAxialLoadCellOffset"=w125:sgl[], "BackupLateralLoadCellOffset"=w124:sgl[], "BackupAxialLoadCellSensitivity"=w123:sgl[], "BackupLateralLoadCellSensitivity"=w122:sgl[], "DCAAxialGain"=w121:sgl[], "DCALateralGain"=w120:sgl[], "DCAUniqueId"=w119:i64[], "DCAFirmwareType"=w118:u8[], "DCAMajorRevision"=w117:u8[], "DCAMinorRevision"=w116:u8[], "MainCalibrationError"=w150:bool[], "BackupCalibrationError"=w156:bool[], "DCAFirmwareUpdate"=w148:bool[], "UniqueIdCRCError"=w155:bool[], "ApplicationTypeMismatch"=w146:bool[], "ApplicationMissing"=w154:bool[], "ApplicationCRCMismatch"=w144:bool[], "OneWireMissing"=w153:bool[], "OneWire1Mismatch"=w142:bool[], "OneWire2Mismatch"=w152:bool[], "DCAUniqueIdCRCError"=w140:bool[], "DCAMainCalibrationError"=w151:bool[], "DCABackupCalibrationError"=w138:bool[])  [unwired: 1 in, 4 out]
        n74 = Not(x=w151) -> (.not. x?=w139:bool[])
        n75 = for {
          N: 156 -> [_]
          tunnel: [w276] -> w240 mode=indexing
          i -> [w277]
          n76 = To Unsigned Byte Integer(number=w277) -> (unsigned 8bit integer=w276:u8)
        }
        n77 = Not(x=w152) -> (.not. x?=w141:bool[])
        n78 = Equal?(x=w212, y=T3 1.0) -> (x = y?=w210:bool)
        n79 = Not(x=w156) -> (.not. x?=w149:bool[])
        n80 = Not(x=w154) -> (.not. x?=w145:bool[])
        n81 = Not(x=w155) -> (.not. x?=w147:bool[])
        n82 = Not(x=w153) -> (.not. x?=w143:bool[])
        n83 = Add(x=w240, y=2) -> (x+y=w238:i32[])
        n84 = Add(x=w240, y=sgl 3.0) -> (x+y=w237:sgl[])
        n85 = Add(x=w240, y=sgl 4.0) -> (x+y=w235:sgl[])
        n86 = Add(x=w240, y=sgl 5.0) -> (x+y=w233:sgl[])
        n87 = Add(x=w240, y=i64 6) -> (x+y=w231:i64[])
        n88 = Add(x=w240, y=u8 7) -> (x+y=w229:u8[])
        n89 = Add(x=w240, y=u8 8) -> (x+y=w227:u8[])
        n90 = Add(x=w240, y=u8 9) -> (x+y=w225:u8[])
        n91 = Add(x=w240, y=u8 10) -> (x+y=w223:u8[])
        n92 = Add(x=w240, y=u8 11) -> (x+y=w221:u8[])
        n93 = Add(x=w240, y=u8 12) -> (x+y=w219:u8[])
        n94 = Add(x=w240, y=u8 13) -> (x+y=w217:u8[])
        n95 = Add(x=w240, y=sgl 14.0) -> (x+y=w200:sgl[])
        n96 = Add(x=w240, y=sgl 15.0) -> (x+y=w199:sgl[])
        n97 = Add(x=w240, y=sgl 16.0) -> (x+y=w198:sgl[])
        n98 = Add(x=w240, y=sgl 17.0) -> (x+y=w197:sgl[])
        n99 = Add(x=w240, y=sgl 18.0) -> (x+y=w196:sgl[])
        n100 = Add(x=w240, y=sgl 19.0) -> (x+y=w195:sgl[])
        n101 = Add(x=w240, y=sgl 20.0) -> (x+y=w194:sgl[])
        n102 = Add(x=w240, y=sgl 21.0) -> (x+y=w193:sgl[])
        n103 = Add(x=w240, y=sgl 22.0) -> (x+y=w192:sgl[])
        n104 = Add(x=w240, y=sgl 23.0) -> (x+y=w191:sgl[])
        n105 = Add(x=w240, y=sgl 24.0) -> (x+y=w169:sgl[])
        n106 = Add(x=w240, y=sgl 25.0) -> (x+y=w190:sgl[])
        n107 = Add(x=w240, y=sgl 26.0) -> (x+y=w189:sgl[])
        n108 = Add(x=w240, y=sgl 27.0) -> (x+y=w188:sgl[])
        n109 = Add(x=w240, y=sgl 28.0) -> (x+y=w187:sgl[])
        n110 = Add(x=w240, y=sgl 29.0) -> (x+y=w186:sgl[])
        n111 = Add(x=w240, y=sgl 30.0) -> (x+y=w185:sgl[])
        n112 = Add(x=w240, y=sgl 31.0) -> (x+y=w184:sgl[])
        n113 = Add(x=w240, y=i64 32) -> (x+y=w183:i64[])
        n114 = Add(x=w240, y=u8 33) -> (x+y=w182:u8[])
        n115 = Add(x=w240, y=u8 34) -> (x+y=w181:u8[])
        n116 = Add(x=w240, y=u8 35) -> (x+y=w180:u8[])
        n117 = Equal?(x=w239, y=w238) -> (x = y?=w215:bool[])
        n118 = Equal?(x=w236, y=w237) -> (x = y?=w214:bool[])
        n119 = Equal?(x=w234, y=w235) -> (x = y?=w213:bool[])
        n120 = Equal?(x=w232, y=w233) -> (x = y?=w209:bool[])
        n121 = Equal?(x=w230, y=w231) -> (x = y?=w208:bool[])
        n122 = Equal?(x=w228, y=w229) -> (x = y?=w207:bool[])
        n123 = Equal?(x=w226, y=w227) -> (x = y?=w206:bool[])
        n124 = Equal?(x=w224, y=w225) -> (x = y?=w205:bool[])
        n125 = Equal?(x=w222, y=w223) -> (x = y?=w204:bool[])
        n126 = Equal?(x=w220, y=w221) -> (x = y?=w203:bool[])
        n127 = Equal?(x=w218, y=w219) -> (x = y?=w202:bool[])
        n128 = Equal?(x=w216, y=w217) -> (x = y?=w201:bool[])
        n129 = Equal?(x=w137, y=w200) -> (x = y?=w179:bool[])
        n130 = Equal?(x=w136, y=w199) -> (x = y?=w178:bool[])
        n131 = Equal?(x=w135, y=w198) -> (x = y?=w177:bool[])
        n132 = Equal?(x=w134, y=w197) -> (x = y?=w176:bool[])
        n133 = Equal?(x=w133, y=w196) -> (x = y?=w175:bool[])
        n134 = Equal?(x=w132, y=w195) -> (x = y?=w174:bool[])
        n135 = Equal?(x=w131, y=w194) -> (x = y?=w173:bool[])
        n136 = Equal?(x=w130, y=w193) -> (x = y?=w172:bool[])
        n137 = Equal?(x=w129, y=w192) -> (x = y?=w171:bool[])
        n138 = Equal?(x=w128, y=w191) -> (x = y?=w170:bool[])
        n139 = Equal?(x=w127, y=w169) -> (x = y?=w168:bool[])
        n140 = Equal?(x=w126, y=w190) -> (x = y?=w167:bool[])
        n141 = Equal?(x=w125, y=w189) -> (x = y?=w166:bool[])
        n142 = Equal?(x=w124, y=w188) -> (x = y?=w165:bool[])
        n143 = Equal?(x=w123, y=w187) -> (x = y?=w164:bool[])
        n144 = Equal?(x=w122, y=w186) -> (x = y?=w163:bool[])
        n145 = Equal?(x=w121, y=w185) -> (x = y?=w162:bool[])
        n146 = Equal?(x=w120, y=w184) -> (x = y?=w161:bool[])
        n147 = Equal?(x=w119, y=w183) -> (x = y?=w160:bool[])
        n148 = Equal?(x=w118, y=w182) -> (x = y?=w159:bool[])
        n149 = Equal?(x=w117, y=w181) -> (x = y?=w158:bool[])
        n150 = Equal?(x=w116, y=w180) -> (x = y?=w157:bool[])
        n151 = Compound Arithmetic op=AND(w210, w215, w214, w213, w209, w208, w207, w206, w205, w204, w203, w202, w201, w179, w178, w177, w176, w175, w174, w173, w172, w171, w170, w168, w167, w166, w165, w164, w163, w162, w161, w160, w159, w158, w157, w150, w149, w148, w147, w146, w145, w144, w143, w142, w141, w140, w139, w138) -> (w115:bool[])
        n152 = And Array Elements(Boolean array=w115) -> (logical AND=→"ForceActuatorInfo":bool)
      }
      event User Event {
        n153 = event-data() -> ("Timestamp"=w304:T3, "AllInSafetyLimit"=w301:bool, "SafetyLimitOk"=w315:bool[], "MirrorWeightOk"=w299:bool, "XMomentOk"=w314:bool, "YMomentOk"=w297:bool, "AllNeighborsOk"=w313:bool, "NeighborsOk"=w295:bool[], "MagnitudeOk"=w312:bool, "AllGlobalBendingOk"=w293:bool, "GlobalBendingOk"=w311:bool[], "FollowingErrorOk"=w291:bool, "AxialFollowingErrorOk"=w309:bool[], "LateralFollowingErrorOk"=w289:bool[], "AOSNetForceOk"=w310:bool, "AllElevationForcesOk"=w287:bool, "ElevationForcesOk"=w308:bool[], "AllAzimuthForcesOk"=w285:bool, "AzimuthForcesOk"=w307:bool[], "AllThermalForcesOk"=w283:bool, "ThermalForcesOk"=w306:bool[], "AllAOSForcesOk"=w281:bool, "AOSForcesOk"=w305:bool[])  [unwired: 1 in, 4 out]
        n154 = Not(x=w315) -> (.not. x?=w300:bool[])
        n155 = Not(x=w314) -> (.not. x?=w298:bool)
        n156 = Not(x=w313) -> (.not. x?=w296:bool)
        n157 = Not(x=w312) -> (.not. x?=w294:bool)
        n158 = Not(x=w311) -> (.not. x?=w292:bool[])
        n159 = Not(x=w309) -> (.not. x?=w290:bool[])
        n160 = Not(x=w310) -> (.not. x?=w288:bool)
        n161 = Not(x=w308) -> (.not. x?=w286:bool[])
        n162 = Not(x=w307) -> (.not. x?=w284:bool[])
        n163 = Not(x=w306) -> (.not. x?=w282:bool[])
        n164 = Not(x=w305) -> (.not. x?=w280:bool[])
        n165 = Equal?(x=w304, y=T3 1.0) -> (x = y?=w302:bool)
        n166 = Compound Arithmetic op=AND(w302, w301, w300, w299, w298, w297, w296, w295, w294, w293, w292, w291, w290, w289, w288, w287, w286, w285, w284, w283, w282, w281, w280) -> (w279:bool[])
        n167 = And Array Elements(Boolean array=w279) -> (logical AND=→"ForceActuatorSafetyChecks":bool)
      }
      event User Event {
        n168 = event-data() -> ("Timestamp"=w325:T3, "ActuatorId"=w323:i32, "TestStatus"=w321:T5)  [unwired: 1 in, 4 out]
        n169 = Equal?(x=w323, y=2) -> (x = y?=w318:bool)
        n170 = Equal?(x=w321, y=TestStatus."Pass") -> (x = y?=w317:bool)
        n171 = Equal?(x=w325, y=T3 1.0) -> (x = y?=w319:bool)
        n172 = Compound Arithmetic op=AND(w319, w318, w317) -> (→"ForceActuatorTest":bool)
      }
      event User Event {
        n173 = event-data() -> ("Timestamp"=w333:T3, "ActuatorId"=w331:i32, "ForceOk"=w329:bool)  [unwired: 1 in, 4 out]
        n174 = Equal?(x=w333, y=T3 1.0) -> (x = y?=w327:bool)
        n175 = Equal?(x=w331, y=2) -> (x = y?=w328:bool)
        n176 = Compound Arithmetic op=AND(w327, w328, w329) -> (→"HardpointActuatorBreakaway":bool)
      }
      event User Event {
        n177 = event-data() -> ("Timestamp"=w341:T3, "ActuatorId"=w339:i32, "Chasing"=w337:bool)  [unwired: 1 in, 4 out]
        n178 = Equal?(x=w341, y=T3 1.0) -> (x = y?=w335:bool)
        n179 = Equal?(x=w339, y=2) -> (x = y?=w336:bool)
        n180 = Compound Arithmetic op=AND(w335, w336, w337) -> (→"HardpointActuatorChase":bool)
      }
      event User Event {
        n181 = event-data() -> ("Timestamp"=w410:T7, "ReferenceId"=w369:i32[], "ReferencePosition"=w368:i32[], "XPosition"=w367:sgl[], "YPosition"=w366:sgl[], "ZPosition"=w365:sgl[], "ILCUniqueId"=w364:i64[], "ILCApplicationType"=w363:u8[], "NetworkNodeType"=w362:u8[], "ILCSelectedOptions"=w361:u8[], "NetworkNodeOptions"=w360:u8[], "MajorRevision"=w359:u8[], "MinorRevision"=w358:u8[], "ADCScanRate"=w357:u8[], "MainADCCalibrationK1"=w356:sgl[], "MainADCCalibrationK2"=w355:sgl[], "MainADCCalibrationK3"=w354:sgl[], "MainADCCalibrationK4"=w353:sgl[], "MainLoadCellOffset"=w352:sgl[], "MainLoadCellSensitivity"=w351:sgl[], "BackupADCCalibrationK1"=w350:sgl[], "BackupADCCalibrationK2"=w349:sgl[], "BackupADCCalibrationK3"=w347:sgl[], "BackupADCCalibrationK4"=w346:sgl[], "BackupLoadCellOffset"=w345:sgl[], "BackupLoadCellSensitivity"=w344:sgl[], "MainCalibrationError"=w378:bool[], "BackupCalibrationError"=w382:bool[], "UniqueIdCRCError"=w376:bool[], "ApplicationTypeMismatch"=w381:bool[], "ApplicationMissing"=w374:bool[], "ApplicationCRCMismatch"=w380:bool[], "OneWireMissing"=w372:bool[], "OneWire1Mismatch"=w379:bool[], "OneWire2Mismatch"=w370:bool[])  [unwired: 1 in, 4 out]
        n182 = for {
          N: 6 -> [_]
          tunnel: [w464] -> w435 mode=indexing
          tunnel: [TRUE] -> _ mode=indexing
          tunnel: [FALSE] -> _ mode=indexing
          i -> [w465]
          n183 = To Unsigned Byte Integer(number=w465) -> (unsigned 8bit integer=w464:u8)
        }
        n184 = Equal?(x=w410, y=T3 1.0) -> (x = y?=w408:bool)
        n185 = Not(x=w382) -> (.not. x?=w377:bool[])
        n186 = Not(x=w380) -> (.not. x?=w373:bool[])
        n187 = Not(x=w381) -> (.not. x?=w375:bool[])
        n188 = Not(x=w379) -> (.not. x?=w371:bool[])
        n189 = Add(x=w435, y=2) -> (x+y=w434:i32[])
        n190 = Add(x=w435, y=3) -> (x+y=w433:i32[])
        n191 = Add(x=w435, y=sgl 4.0) -> (x+y=w432:sgl[])
        n192 = Add(x=w435, y=sgl 5.0) -> (x+y=w431:sgl[])
        n193 = Add(x=w435, y=sgl 6.0) -> (x+y=w430:sgl[])
        n194 = Add(x=w435, y=i64 7) -> (x+y=w429:i64[])
        n195 = Add(x=w435, y=u8 8) -> (x+y=w428:u8[])
        n196 = Add(x=w435, y=u8 9) -> (x+y=w427:u8[])
        n197 = Add(x=w435, y=u8 10) -> (x+y=w426:u8[])
        n198 = Add(x=w435, y=u8 11) -> (x+y=w425:u8[])
        n199 = Add(x=w435, y=u8 12) -> (x+y=w424:u8[])
        n200 = Add(x=w435, y=u8 13) -> (x+y=w423:u8[])
        n201 = Add(x=w435, y=u8 14) -> (x+y=w422:u8[])
        n202 = Add(x=w435, y=sgl 15.0) -> (x+y=w421:sgl[])
        n203 = Add(x=w435, y=sgl 16.0) -> (x+y=w420:sgl[])
        n204 = Add(x=w435, y=sgl 17.0) -> (x+y=w419:sgl[])
        n205 = Add(x=w435, y=sgl 18.0) -> (x+y=w418:sgl[])
        n206 = Add(x=w435, y=sgl 19.0) -> (x+y=w417:sgl[])
        n207 = Add(x=w435, y=sgl 20.0) -> (x+y=w416:sgl[])
        n208 = Add(x=w435, y=sgl 21.0) -> (x+y=w415:sgl[])
        n209 = Add(x=w435, y=sgl 22.0) -> (x+y=w414:sgl[])
        n210 = Add(x=w435, y=sgl 23.0) -> (x+y=w348:sgl[])
        n211 = Add(x=w435, y=sgl 24.0) -> (x+y=w413:sgl[])
        n212 = Add(x=w435, y=sgl 25.0) -> (x+y=w412:sgl[])
        n213 = Add(x=w435, y=sgl 26.0) -> (x+y=w411:sgl[])
        n214 = Equal?(x=w369, y=w434) -> (x = y?=w407:bool[])
        n215 = Equal?(x=w368, y=w433) -> (x = y?=w406:bool[])
        n216 = Equal?(x=w367, y=w432) -> (x = y?=w405:bool[])
        n217 = Equal?(x=w366, y=w431) -> (x = y?=w404:bool[])
        n218 = Equal?(x=w365, y=w430) -> (x = y?=w403:bool[])
        n219 = Equal?(x=w364, y=w429) -> (x = y?=w402:bool[])
        n220 = Equal?(x=w363, y=w428) -> (x = y?=w401:bool[])
        n221 = Equal?(x=w362, y=w427) -> (x = y?=w400:bool[])
        n222 = Equal?(x=w361, y=w426) -> (x = y?=w399:bool[])
        n223 = Equal?(x=w360, y=w425) -> (x = y?=w398:bool[])
        n224 = Equal?(x=w359, y=w424) -> (x = y?=w397:bool[])
        n225 = Equal?(x=w358, y=w423) -> (x = y?=w396:bool[])
        n226 = Equal?(x=w357, y=w422) -> (x = y?=w395:bool[])
        n227 = Equal?(x=w356, y=w421) -> (x = y?=w394:bool[])
        n228 = Equal?(x=w355, y=w420) -> (x = y?=w393:bool[])
        n229 = Equal?(x=w354, y=w419) -> (x = y?=w392:bool[])
        n230 = Equal?(x=w353, y=w418) -> (x = y?=w391:bool[])
        n231 = Equal?(x=w352, y=w417) -> (x = y?=w390:bool[])
        n232 = Equal?(x=w351, y=w416) -> (x = y?=w389:bool[])
        n233 = Equal?(x=w350, y=w415) -> (x = y?=w388:bool[])
        n234 = Equal?(x=w349, y=w414) -> (x = y?=w387:bool[])
        n235 = Equal?(x=w347, y=w348) -> (x = y?=w386:bool[])
        n236 = Equal?(x=w346, y=w413) -> (x = y?=w385:bool[])
        n237 = Equal?(x=w345, y=w412) -> (x = y?=w384:bool[])
        n238 = Equal?(x=w344, y=w411) -> (x = y?=w383:bool[])
        n239 = Compound Arithmetic op=AND(w408, w407, w406, w405, w404, w403, w402, w401, w400, w399, w398, w397, w396, w395, w394, w393, w392, w391, w390, w389, w388, w387, w386, w385, w384, w383, w378, w377, w376, w375, w374, w373, w372, w371, w370) -> (w343:bool[])
        n240 = And Array Elements(Boolean array=w343) -> (logical AND=→"HardpointActuatorInfo":bool)
      }
      event User Event {
        n241 = event-data() -> ("Timestamp"=w473:T3, "ActuatorId"=w471:i32, "CommunicationOK"=w469:bool)  [unwired: 1 in, 4 out]
        n242 = Equal?(x=w473, y=T3 1.0) -> (x = y?=w467:bool)
        n243 = Equal?(x=w471, y=2) -> (x = y?=w468:bool)
        n244 = Compound Arithmetic op=AND(w467, w468, w469) -> (→"ILCCommunication":bool)
      }
      event User Event {
        n245 = event-data() -> ("Timestamp"=w478:T3, "Successful"=w475:bool)  [unwired: 1 in, 4 out]
        n246 = Equal?(x=w478, y=T3 1.0) -> (x = y?=w476:bool)
        n247 = Compound Arithmetic op=AND(w476, w475) -> (→"LowerMirrorComplete":bool)
      }
      event User Event {
        n248 = event-data() -> ("Timestamp"=w481:T3, "Successful"=w480:bool)  [unwired: 1 in, 4 out]
        n249 = Equal?(x=w481, y=T3 1.0) -> (x = y?=w482:bool)
        n250 = Compound Arithmetic op=AND(w482, w480) -> (→"RaiseMirrorComplete":bool)
      }
      event User Event {
        n251 = event-data() -> ("Timestamp"=w489:T3, "HardpointChase"=w488:bool, "HardpointOffloading"=w487:bool, "OuterLoopTimeOk"=w485:bool)  [unwired: 1 in, 4 out]
        n252 = Not(x=w487) -> (.not. x?=w486:bool)
        n253 = Equal?(x=w489, y=T3 1.0) -> (x = y?=w490:bool)
        n254 = Compound Arithmetic op=AND(w490, w488, w486, w485) -> (→"ServoLoops":bool)
      }
      event User Event {
        n255 = event-data() -> ("Timestamp"=w496:T3, "Settings"=w495:string)  [unwired: 1 in, 4 out]
        n256 = Equal?(x=w496, y=T3 1.0) -> (x = y?=w497:bool)
        n257 = Equal?(x=w495, y="Two") -> (x = y?=w493:bool)
        n258 = Compound Arithmetic op=AND(w497, w493) -> (→"SettingsApplied":bool)
      }
      event User Event {
        n259 = event-data() -> ("Timestamp"=w503:T3, "RecommendedSettingsVersion"=w502:string)  [unwired: 1 in, 4 out]
        n260 = Equal?(x=w503, y=T3 1.0) -> (x = y?=w504:bool)
        n261 = Equal?(x=w502, y="Two") -> (x = y?=w500:bool)
        n262 = Compound Arithmetic op=AND(w504, w500) -> (→"SettingVersions":bool)
      }
      event User Event {
        n263 = event-data() -> ("Timestamp"=w516:T3, "ILCVersionsOk"=w514:bool, "DCAVersionsOk"=w515:bool, "ILCFirmwareOk"=w512:bool, "DCAFirmwareOk"=w511:bool, "ILCStatusOk"=w508:bool, "DCAStatusOk"=w510:bool)  [unwired: 1 in, 4 out]
        n264 = Not(x=w515) -> (.not. x?=w513:bool)
        n265 = Not(x=w511) -> (.not. x?=w509:bool)
        n266 = Not(x=w510) -> (.not. x?=w507:bool)
        n267 = Equal?(x=w516, y=T3 1.0) -> (x = y?=w517:bool)
        n268 = Compound Arithmetic op=AND(w517, w514, w513, w512, w509, w508, w507) -> (→"StartupChecks":bool)
      }
      event User Event {
        n269 = event-data() -> ("Timestamp"=w526:T3, "ILCResetOk"=w523:bool, "DCAResetOk"=w525:bool, "ILCPowerOk"=w521:bool, "DCAPowerOk"=w524:bool)  [unwired: 1 in, 4 out]
        n270 = Not(x=w525) -> (.not. x?=w522:bool)
        n271 = Not(x=w524) -> (.not. x?=w520:bool)
        n272 = Equal?(x=w526, y=T3 1.0) -> (x = y?=w527:bool)
        n273 = Compound Arithmetic op=AND(w527, w523, w522, w521, w520) -> (→"StatusChecks":bool)
      }
      event User Event {
        n274 = event-data() -> ("Timestamp"=w533:T7, "SummaryStates"=w532:T8)  [unwired: 1 in, 4 out]
        n275 = Equal?(x=w533, y=T3 1.0) -> (x = y?=w534:bool)
        n276 = Equal?(x=w532, y=SummaryStates."DisabledState" ("SummaryStates")) -> (x = y?=w531:bool)
        n277 = Compound Arithmetic op=AND(w534, w531) -> (→"SummaryState":bool)
      }
    }
  }
  n278 = call-dynamic "startClient.vi"("error in (no error)"=w44, "M1M3SAL in"=w46) -> ("error out"=w35:errorcluster, "M1M3SAL out"=w41:refnum<class "M1M3SAL.lvclass">)  [unwired: 8 in]
  n279 = call-dynamic "run.vi"("error in (no error)"=w35, "M1M3SAL in"=w41) -> ()  [unwired: 8 in, 2 out]
  n280 = flat-sequence {
    tunnel: w35 -> [_]
    frame #0 {
      n281 = local write "Ready?"(TRUE ("Ready?")) -> ()
    }
  }
  n282 = while {
    shift-right: [w540] -> w40
    shift-left: w41 -> [w541]
    shift-right: [w538] -> w43
    shift-left: w35 -> [w539]
    stop <- w537 stop-if-true
    n283 = event shown="[10] \"HardpointActuatorInfoGo\": Value Change" {
      selector: _ -> [_ _ _ _ _ _ _ _ _ _ _ _ _ _ _ _ _ _ _ _ _ _ _ _]
      dyn-events: _ -> [_ _ _ _ _ _ _ _ _ _ _ _ _ _ _ _ _ _ _ _ _ _ _ _]
      timeout: _ -> [_ _ _ _ _ _ _ _ _ _ _ _ _ _ _ _ _ _ _ _ _ _ _ _]
      tunnel: w541 -> [w546 w551 w556 w561 w566 w571 w576 w588 w595 w672 w697 w747 w753 w758 w763 w768 w773 w778 w783 w788 w793 w798 w803 w805]
      tunnel: [w545 w550 w552 w560 w565 w570 w575 w587 w594 w669 w694 w745 w751 w755 w760 w765 w770 w777 w782 w784 w790 w795 w801 w805] -> w540
      tunnel: w539 -> [w543 w548 w554 w558 w563 w568 w573 w585 w592 w671 w695 w746 w752 w757 w761 w766 w771 w775 w780 w786 w792 w797 w799 w804]
      tunnel: [w544 w549 w553 w559 w564 w569 w574 w586 w593 w670 w693 w744 w750 w754 w759 w764 w769 w776 w781 w785 w791 w794 w800 w804] -> w538
      tunnel: [_ _ _ _ _ _ _ _ _ _ _ _ _ _ _ _ _ _ _ _ _ _ _ w806] -> w537
      event "ActuatorBroadcastCounterGo": Value Change {
        n284 = event-data() -> ()  [unwired: 1 in, 3 out]
        n285 = call-dynamic "logActuatorBroadcastCounter.vi"("error in (no error)"=w543, "EventActuatorBroadcastCounter"=T9 {"Timestamp"=1.0, "ActuatorId"=2, "CounterOk"=TRUE}, "M1M3SAL in"=w546) -> ("error out"=w544:errorcluster, "M1M3SAL out"=w545:refnum<class "M1M3SAL.lvclass">)  [unwired: 7 in]
      }
      event "ActuatorTestStatusGo": Value Change {
        n286 = event-data() -> ()  [unwired: 1 in, 3 out]
        n287 = call-dynamic "logActuatorTestStatus.vi"("error in (no error)"=w548, "EventActuatorTestStatus"=T10 {"Timestamp"=1.0, "AllTestsRan"=TRUE}, "M1M3SAL in"=w551) -> ("error out"=w549:errorcluster, "M1M3SAL out"=w550:refnum<class "M1M3SAL.lvclass">)  [unwired: 7 in]
      }
      event "AirStatusGo": Value Change {
        n288 = event-data() -> ()  [unwired: 1 in, 3 out]
        n289 = call-dynamic "logAirStatus.vi"("error in (no error)"=w554, "EventAirStatus"=T11 {"Timestamp"=1.0, "AirCommandedOn"=TRUE, "AirOn"=FALSE, "AirPressureOk"=TRUE, "HardpointAirPressureOk"=FALSE}, "M1M3SAL in"=w556) -> ("error out"=w553:errorcluster, "M1M3SAL out"=w552:refnum<class "M1M3SAL.lvclass">)  [unwired: 7 in]
      }
      event "AppliedSettingsMatchStartGo": Value Change {
        n290 = event-data() -> ()  [unwired: 1 in, 3 out]
        n291 = call-dynamic "logAppliedSettingsMatchStart.vi"("error in (no error)"=w558, "EventAppliedSettingsMatchStart"=T12 {"Timestamp"=1.0, "AppliedSettingsMatchStart"=TRUE}, "M1M3SAL in"=w561) -> ("error out"=w559:errorcluster, "M1M3SAL out"=w560:refnum<class "M1M3SAL.lvclass">)  [unwired: 7 in]
      }
      event "CellChecksGo": Value Change {
        n292 = event-data() -> ()  [unwired: 1 in, 3 out]
        n293 = call-dynamic "logCellChecks.vi"("error in (no error)"=w563, "EventCellChecks"=T13 {"Timestamp"=1.0, "MirrorDoorClosed"=TRUE}, "M1M3SAL in"=w566) -> ("error out"=w564:errorcluster, "M1M3SAL out"=w565:refnum<class "M1M3SAL.lvclass">)  [unwired: 7 in]
      }
      event "DetailedStateGo": Value Change {
        n294 = event-data() -> ()  [unwired: 1 in, 3 out]
        n295 = call-dynamic "logDetailedState.vi"("error in (no error)"=w568, "EventDetailedState"=T14 {"Timestamp"=1.0, "DetailedStates"=enum."StandbyState"}, "M1M3SAL in"=w571) -> ("error out"=w569:errorcluster, "M1M3SAL out"=w570:refnum<class "M1M3SAL.lvclass">)  [unwired: 7 in]
      }
      event "ElevationAngleChecksGo": Value Change {
        n296 = event-data() -> ()  [unwired: 1 in, 6 out]
        n297 = call-dynamic "logElevationAngleChecks.vi"("error in (no error)"=w573, "EventElevationAngleChecks"=T15 {"Timestamp"=1.0, "MatchesTMA"=TRUE, "MatchesInclinometer"=FALSE, "MatchesMeasured"=TRUE}, "M1M3SAL in"=w576) -> ("error out"=w574:errorcluster, "M1M3SAL out"=w575:refnum<class "M1M3SAL.lvclass">)  [unwired: 7 in]
      }
      event "ForceActuatorSafetyChecksGo": Value Change {
        w579 = FALSE ("MirrorWeightOk")
        w578 = TRUE ("AllInSafetyLimit")
        n298 = event-data() -> ()  [unwired: 1 in, 6 out]
        n299 = for {
          N: 156 -> [_]
          tunnel: [TRUE ("AllInSafetyLimit")] -> w580 mode=indexing
          tunnel: [FALSE ("AllInSafetyLimit")] -> w577 mode=indexing
        }
        n300 = Bundle By Name(cluster=T16 {"Timestamp"=0.0, "AllInSafetyLimit"=FALSE, "SafetyLimitOk"=[], "MirrorWeightOk"=FALSE, "XMomentOk"=FALSE, "YMomentOk"=FALSE, "AllNeighborsOk"=FALSE, "NeighborsOk"=[], "MagnitudeOk"=FALSE, "AllGlobalBendingOk"=FALSE, "GlobalBendingOk"=[], "FollowingErrorOk"=FALSE, "AxialFollowingErrorOk"=[], "LateralFollowingErrorOk"=[], "AOSNetForceOk"=FALSE, "AllElevationForcesOk"=FALSE, "ElevationForcesOk"=[], "AllAzimuthForcesOk"=FALSE, "AzimuthForcesOk"=[], "AllThermalForcesOk"=FALSE, "ThermalForcesOk"=[], "AllAOSForcesOk"=FALSE, "AOSForcesOk"=[]} ("EventForceActuatorSafetyChecks"), "Timestamp"=T3 1.0, "AllInSafetyLimit"=w578, "SafetyLimitOk"=w577, "MirrorWeightOk"=w578, "XMomentOk"=w579, "YMomentOk"=w578, "AllNeighborsOk"=w579, "NeighborsOk"=w580, "MagnitudeOk"=w579, "AllGlobalBendingOk"=w578, "GlobalBendingOk"=w577, "FollowingErrorOk"=w578, "AxialFollowingErrorOk"=w577, "LateralFollowingErrorOk"=w580, "AOSNetForceOk"=w579, "AllElevationForcesOk"=w578, "ElevationForcesOk"=w577, "AllAzimuthForcesOk"=w578, "AzimuthForcesOk"=w577, "AllThermalForcesOk"=w578, "ThermalForcesOk"=w577, "AllAOSForcesOk"=w578, "AOSForcesOk"=w577) -> (w583:T16)
        n301 = call-dynamic "logForceActuatorSafetyCheck.vi"("error in (no error)"=w585, "EventForceActuatorSafetyChecks"=w583, "M1M3SAL in"=w588) -> ("error out"=w586:errorcluster, "M1M3SAL out"=w587:refnum<class "M1M3SAL.lvclass">)  [unwired: 7 in]
      }
      event "ErrorCodeGo": Value Change {
        n302 = event-data() -> ()  [unwired: 1 in, 6 out]
        n303 = call-dynamic "logErrorCode.vi"("error in (no error)"=w592, "EventErrorCode"=T17 {"Timestamp"=1.0, "ErrorCode"=2}, "M1M3SAL in"=w595) -> ("error out"=w593:errorcluster, "M1M3SAL out"=w594:refnum<class "M1M3SAL.lvclass">)  [unwired: 7 in]
      }
      event "ForceActuatorInfoGo": Value Change {
        n304 = event-data() -> ()  [unwired: 1 in, 6 out]
        n305 = for {
          N: 156 -> [_]
          tunnel: [w677] -> w600 mode=indexing
          tunnel: [TRUE] -> w597 mode=indexing
          tunnel: [FALSE] -> w596 mode=indexing
          i -> [w678]
          n306 = To Unsigned Byte Integer(number=w678) -> (unsigned 8bit integer=w677:u8)
        }
        n307 = Add(x=w600, y=2) -> (x+y=w665:i32[])
        n308 = Add(x=w600, y=sgl 3.0) -> (x+y=w663:sgl[])
        n309 = Add(x=w600, y=sgl 4.0) -> (x+y=w661:sgl[])
        n310 = Add(x=w600, y=sgl 5.0) -> (x+y=w659:sgl[])
        n311 = Add(x=w600, y=i64 6) -> (x+y=w657:i64[])
        n312 = Add(x=w600, y=u8 7) -> (x+y=w655:u8[])
        n313 = Add(x=w600, y=u8 8) -> (x+y=w653:u8[])
        n314 = Add(x=w600, y=u8 9) -> (x+y=w651:u8[])
        n315 = Add(x=w600, y=u8 10) -> (x+y=w649:u8[])
        n316 = Add(x=w600, y=u8 11) -> (x+y=w647:u8[])
        n317 = Add(x=w600, y=u8 12) -> (x+y=w645:u8[])
        n318 = Add(x=w600, y=u8 13) -> (x+y=w643:u8[])
        n319 = Add(x=w600, y=sgl 14.0) -> (x+y=w639:sgl[])
        n320 = Add(x=w600, y=sgl 15.0) -> (x+y=w638:sgl[])
        n321 = Add(x=w600, y=sgl 16.0) -> (x+y=w637:sgl[])
        n322 = Add(x=w600, y=sgl 17.0) -> (x+y=w633:sgl[])
        n323 = Add(x=w600, y=sgl 18.0) -> (x+y=w632:sgl[])
        n324 = Add(x=w600, y=sgl 19.0) -> (x+y=w631:sgl[])
        n325 = Add(x=w600, y=sgl 20.0) -> (x+y=w620:sgl[])
        n326 = Add(x=w600, y=sgl 21.0) -> (x+y=w619:sgl[])
        n327 = Add(x=w600, y=sgl 22.0) -> (x+y=w618:sgl[])
        n328 = Add(x=w600, y=sgl 23.0) -> (x+y=w617:sgl[])
        n329 = Add(x=w600, y=sgl 24.0) -> (x+y=w616:sgl[])
        n330 = Add(x=w600, y=sgl 25.0) -> (x+y=w615:sgl[])
        n331 = Add(x=w600, y=sgl 26.0) -> (x+y=w614:sgl[])
        n332 = Add(x=w600, y=sgl 27.0) -> (x+y=w613:sgl[])
        n333 = Add(x=w600, y=sgl 28.0) -> (x+y=w612:sgl[])
        n334 = Add(x=w600, y=sgl 29.0) -> (x+y=w608:sgl[])
        n335 = Add(x=w600, y=sgl 30.0) -> (x+y=w607:sgl[])
        n336 = Add(x=w600, y=sgl 31.0) -> (x+y=w606:sgl[])
        n337 = Add(x=w600, y=i64 32) -> (x+y=w605:i64[])
        n338 = Add(x=w600, y=u8 33) -> (x+y=w603:u8[])
        n339 = Add(x=w600, y=u8 34) -> (x+y=w599:u8[])
        n340 = Add(x=w600, y=u8 35) -> (x+y=w598:u8[])
        n341 = Bundle By Name(cluster=T18 {"Timestamp"=0.0, "ReferenceId"=[], "XPosition"=[], "YPosition"=[], "ZPosition"=[], "ILCUniqueId"=[], "ILCApplicationType"=[], "NetworkNodeType"=[], "ILCSelectedOptions"=[], "NetworkNodeOptions"=[], "MajorRevision"=[], "MinorRevision"=[], "ADCScanRate"=[], "MainADCCalibrationK1"=[], "MainADCCalibrationK2"=[], "MainADCCalibrationK3"=[], "MainADCCalibrationK4"=[], "MainAxialLoadCellOffset"=[], "MainLateralLoadCellOffset"=[], "MainAxialLoadCellSensitivity"=[], "MainLateralLoadCellSensitivity"=[], "BackupADCCalibrationK1"=[], "BackupADCCalibrationK2"=[], "BackupADCCalibrationK3"=[], "BackupADCCalibrationK4"=[], "BackupAxialLoadCellOffset"=[], "BackupLateralLoadCellOffset"=[], "BackupAxialLoadCellSensitivity"=[], "BackupLateralLoadCellSensitivity"=[], "DCAAxialGain"=[], "DCALateralGain"=[], "DCAUniqueId"=[], "DCAFirmwareType"=[], "DCAMajorRevision"=[], "DCAMinorRevision"=[], "MainCalibrationError"=[], "BackupCalibrationError"=[], "DCAFirmwareUpdate"=[], "UniqueIdCRCError"=[], "ApplicationTypeMismatch"=[], "ApplicationMissing"=[], "ApplicationCRCMismatch"=[], "OneWireMissing"=[], "OneWire1Mismatch"=[], "OneWire2Mismatch"=[], "DCAUniqueIdCRCError"=[], "DCAMainCalibrationError"=[], "DCABackupCalibrationError"=[], "DCAApplicationMissing"=[], "DCAApplicationCRCMismatch"=[], "DCABootloaderActive"=[]} ("EventForceActuatorInfo"), "Timestamp"=T3 1.0, "ReferenceId"=w665, "XPosition"=w663, "YPosition"=w661, "ZPosition"=w659, "ILCUniqueId"=w657, "ILCApplicationType"=w655, "NetworkNodeType"=w653, "ILCSelectedOptions"=w651, "NetworkNodeOptions"=w649, "MajorRevision"=w647, "MinorRevision"=w645, "ADCScanRate"=w643, "MainADCCalibrationK1"=w639, "MainADCCalibrationK2"=w638, "MainADCCalibrationK3"=w637, "MainADCCalibrationK4"=w633, "MainAxialLoadCellOffset"=w632, "MainLateralLoadCellOffset"=w631, "MainAxialLoadCellSensitivity"=w620, "MainLateralLoadCellSensitivity"=w619, "BackupADCCalibrationK1"=w618, "BackupADCCalibrationK2"=w617, "BackupADCCalibrationK3"=w616, "BackupADCCalibrationK4"=w615, "BackupAxialLoadCellOffset"=w614, "BackupLateralLoadCellOffset"=w613, "BackupAxialLoadCellSensitivity"=w612, "BackupLateralLoadCellSensitivity"=w608, "DCAAxialGain"=w607, "DCALateralGain"=w606, "DCAUniqueId"=w605, "DCAFirmwareType"=w603, "DCAMajorRevision"=w599, "DCAMinorRevision"=w598, "MainCalibrationError"=w597, "BackupCalibrationError"=w596, "DCAFirmwareUpdate"=w597, "UniqueIdCRCError"=w596, "ApplicationTypeMismatch"=w597, "ApplicationMissing"=w596, "ApplicationCRCMismatch"=w597, "OneWireMissing"=w596, "OneWire1Mismatch"=w597, "OneWire2Mismatch"=w596, "DCAUniqueIdCRCError"=w597, "DCAMainCalibrationError"=w596, "DCABackupCalibrationError"=w597, "DCAApplicationMissing"=w596, "DCAApplicationCRCMismatch"=w597, "DCABootloaderActive"=w596) -> (w673:T18)
        n342 = call-dynamic "logForceActuatorInfo.vi"("error in (no error)"=w671, "EventForceActuatorInfo"=w673, "M1M3SAL in"=w672) -> ("error out"=w670:errorcluster, "M1M3SAL out"=w669:refnum<class "M1M3SAL.lvclass">)  [unwired: 7 in]
      }
      event "HardpointActuatorInfoGo": Value Change {
        n343 = event-data() -> ()  [unwired: 1 in, 6 out]
        n344 = for {
          N: 6 -> [_]
          tunnel: [w742] -> w687 mode=indexing
          tunnel: [TRUE] -> w689 mode=indexing
          tunnel: [FALSE] -> w688 mode=indexing
          i -> [w743]
          n345 = To Unsigned Byte Integer(number=w743) -> (unsigned 8bit integer=w742:u8)
        }
        n346 = Add(x=w687, y=2) -> (x+y=w736:i32[])
        n347 = Add(x=w687, y=3) -> (x+y=w690:i32[])
        n348 = Add(x=w687, y=sgl 4.0) -> (x+y=w734:sgl[])
        n349 = Add(x=w687, y=sgl 5.0) -> (x+y=w732:sgl[])
        n350 = Add(x=w687, y=sgl 6.0) -> (x+y=w730:sgl[])
        n351 = Add(x=w687, y=i64 7) -> (x+y=w728:i64[])
        n352 = Add(x=w687, y=u8 8) -> (x+y=w726:u8[])
        n353 = Add(x=w687, y=u8 9) -> (x+y=w724:u8[])
        n354 = Add(x=w687, y=u8 10) -> (x+y=w722:u8[])
        n355 = Add(x=w687, y=u8 11) -> (x+y=w720:u8[])
        n356 = Add(x=w687, y=u8 12) -> (x+y=w718:u8[])
        n357 = Add(x=w687, y=u8 13) -> (x+y=w716:u8[])
        n358 = Add(x=w687, y=u8 14) -> (x+y=w714:u8[])
        n359 = Add(x=w687, y=sgl 15.0) -> (x+y=w710:sgl[])
        n360 = Add(x=w687, y=sgl 16.0) -> (x+y=w709:sgl[])
        n361 = Add(x=w687, y=sgl 17.0) -> (x+y=w708:sgl[])
        n362 = Add(x=w687, y=sgl 18.0) -> (x+y=w704:sgl[])
        n363 = Add(x=w687, y=sgl 19.0) -> (x+y=w686:sgl[])
        n364 = Add(x=w687, y=sgl 20.0) -> (x+y=w685:sgl[])
        n365 = Add(x=w687, y=sgl 21.0) -> (x+y=w684:sgl[])
        n366 = Add(x=w687, y=sgl 22.0) -> (x+y=w683:sgl[])
        n367 = Add(x=w687, y=sgl 23.0) -> (x+y=w682:sgl[])
        n368 = Add(x=w687, y=sgl 24.0) -> (x+y=w681:sgl[])
        n369 = Add(x=w687, y=sgl 25.0) -> (x+y=w680:sgl[])
        n370 = Add(x=w687, y=sgl 26.0) -> (x+y=w679:sgl[])
        n371 = Bundle By Name(cluster=T19 {"Timestamp"=0.0, "ReferenceId"=[], "ReferencePosition"=[], "XPosition"=[], "YPosition"=[], "ZPosition"=[], "ILCUniqueId"=[], "ILCApplicationType"=[], "NetworkNodeType"=[], "ILCSelectedOptions"=[], "NetworkNodeOptions"=[], "MajorRevision"=[], "MinorRevision"=[], "ADCScanRate"=[], "MainADCCalibrationK1"=[], "MainADCCalibrationK2"=[], "MainADCCalibrationK3"=[], "MainADCCalibrationK4"=[], "MainLoadCellOffset"=[], "MainLoadCellSensitivity"=[], "BackupADCCalibrationK1"=[], "BackupADCCalibrationK2"=[], "BackupADCCalibrationK3"=[], "BackupADCCalibrationK4"=[], "BackupLoadCellOffset"=[], "BackupLoadCellSensitivity"=[], "MainCalibrationError"=[], "BackupCalibrationError"=[], "UniqueIdCRCError"=[], "ApplicationTypeMismatch"=[], "ApplicationMissing"=[], "ApplicationCRCMismatch"=[], "OneWireMissing"=[], "OneWire1Mismatch"=[], "OneWire2Mismatch"=[]} ("EventHardpointActuatorInfo"), "Timestamp"=T3 1.0, "ReferenceId"=w736, "ReferencePosition"=w690, "XPosition"=w734, "YPosition"=w732, "ZPosition"=w730, "ILCUniqueId"=w728, "ILCApplicationType"=w726, "NetworkNodeType"=w724, "ILCSelectedOptions"=w722, "NetworkNodeOptions"=w720, "MajorRevision"=w718, "MinorRevision"=w716, "ADCScanRate"=w714, "MainADCCalibrationK1"=w710, "MainADCCalibrationK2"=w709, "MainADCCalibrationK3"=w708, "MainADCCalibrationK4"=w704, "MainLoadCellOffset"=w686, "MainLoadCellSensitivity"=w685, "BackupADCCalibrationK1"=w684, "BackupADCCalibrationK2"=w683, "BackupADCCalibrationK3"=w682, "BackupADCCalibrationK4"=w681, "BackupLoadCellOffset"=w680, "BackupLoadCellSensitivity"=w679, "MainCalibrationError"=w689, "BackupCalibrationError"=w688, "UniqueIdCRCError"=w689, "ApplicationTypeMismatch"=w688, "ApplicationMissing"=w689, "ApplicationCRCMismatch"=w688, "OneWireMissing"=w689, "OneWire1Mismatch"=w688, "OneWire2Mismatch"=w689) -> (w696:T19)
        n372 = call-dynamic "logHardpointActuatorInfo.vi"("error in (no error)"=w695, "EventHardpointActuatorInfo"=w696, "M1M3SAL in"=w697) -> ("error out"=w693:errorcluster, "M1M3SAL out"=w694:refnum<class "M1M3SAL.lvclass">)  [unwired: 7 in]
      }
      event "ForceActuatorTestGo": Value Change {
        n373 = event-data() -> ()  [unwired: 1 in, 6 out]
        n374 = call-dynamic "logForceActuatorTest.vi"("error in (no error)"=w746, "EventForceActuatorTest"=T20 {"Timestamp"=1.0, "ActuatorId"=2, "TestStatus"=enum."Pass"}, "M1M3SAL in"=w747) -> ("error out"=w744:errorcluster, "M1M3SAL out"=w745:refnum<class "M1M3SAL.lvclass">)  [unwired: 7 in]
      }
      event "HardpointActuatorBreakawayGo": Value Change {
        n375 = event-data() -> ()  [unwired: 1 in, 6 out]
        n376 = call-dynamic "logHardpointActuatorBreakaway.vi"("error in (no error)"=w752, "EventHardpointActuatorBreakaway"=T21 {"Timestamp"=1.0, "ActuatorId"=2, "ForceOk"=TRUE}, "M1M3SAL in"=w753) -> ("error out"=w750:errorcluster, "M1M3SAL out"=w751:refnum<class "M1M3SAL.lvclass">)  [unwired: 7 in]
      }
      event "HardpointActuatorChaseGo": Value Change {
        n377 = event-data() -> ()  [unwired: 1 in, 6 out]
        n378 = call-dynamic "logHardpointActuatorChase.vi"("error in (no error)"=w757, "EventHardpointActuatorChase"=T22 {"Timestamp"=1.0, "ActuatorId"=2, "Chasing"=TRUE}, "M1M3SAL in"=w758) -> ("error out"=w754:errorcluster, "M1M3SAL out"=w755:refnum<class "M1M3SAL.lvclass">)  [unwired: 7 in]
      }
      event "ILCCommunicationGo": Value Change {
        n379 = event-data() -> ()  [unwired: 1 in, 6 out]
        n380 = call-dynamic "logILCCommunication.vi"("error in (no error)"=w761, "EventILCCommunication"=T23 {"Timestamp"=1.0, "ActuatorId"=2, "CommunicationOK"=TRUE}, "M1M3SAL in"=w763) -> ("error out"=w759:errorcluster, "M1M3SAL out"=w760:refnum<class "M1M3SAL.lvclass">)  [unwired: 7 in]
      }
      event "LowerMirrorCompleteGo": Value Change {
        n381 = event-data() -> ()  [unwired: 1 in, 6 out]
        n382 = call-dynamic "logLowerMirrorComplete.vi"("error in (no error)"=w766, "EventLowerMirrorComplete"=T24 {"Timestamp"=1.0, "Successful"=TRUE}, "M1M3SAL in"=w768) -> ("error out"=w764:errorcluster, "M1M3SAL out"=w765:refnum<class "M1M3SAL.lvclass">)  [unwired: 7 in]
      }
      event "RaiseMirrorCompleteGo": Value Change {
        n383 = event-data() -> ()  [unwired: 1 in, 6 out]
        n384 = call-dynamic "logRaiseMirrorComplete.vi"("error in (no error)"=w771, "EventRaiseMirrorComplete"=T25 {"Timestamp"=1.0, "Successful"=TRUE}, "M1M3SAL in"=w773) -> ("error out"=w769:errorcluster, "M1M3SAL out"=w770:refnum<class "M1M3SAL.lvclass">)  [unwired: 7 in]
      }
      event "ServoLoopsGo": Value Change {
        n385 = event-data() -> ()  [unwired: 1 in, 6 out]
        n386 = call-dynamic "logServoLoops.vi"("error in (no error)"=w775, "EventServoLoops"=T26 {"Timestamp"=1.0, "HardpointChase"=TRUE, "HardpointOffloading"=FALSE, "OuterLoopTimeOk"=TRUE}, "M1M3SAL in"=w778) -> ("error out"=w776:errorcluster, "M1M3SAL out"=w777:refnum<class "M1M3SAL.lvclass">)  [unwired: 7 in]
      }
      event "SettingsAppliedGo": Value Change {
        n387 = event-data() -> ()  [unwired: 1 in, 6 out]
        n388 = call-dynamic "logSettingsApplied.vi"("error in (no error)"=w780, "EventSettingsApplied"=T27 {"Timestamp"=1.0, "Settings"="Two"}, "M1M3SAL in"=w783) -> ("error out"=w781:errorcluster, "M1M3SAL out"=w782:refnum<class "M1M3SAL.lvclass">)  [unwired: 7 in]
      }
      event "SettingVersionsGo": Value Change {
        n389 = event-data() -> ()  [unwired: 1 in, 6 out]
        n390 = call-dynamic "logSettingVersions.vi"("error in (no error)"=w786, "EventSettingVersions"=T28 {"Timestamp"=1.0, "RecommendedSettingsVersion"="Two"}, "M1M3SAL in"=w788) -> ("error out"=w785:errorcluster, "M1M3SAL out"=w784:refnum<class "M1M3SAL.lvclass">)  [unwired: 7 in]
      }
      event "StartupChecksGo": Value Change {
        n391 = event-data() -> ()  [unwired: 1 in, 6 out]
        n392 = call-dynamic "logStartupChecks.vi"("error in (no error)"=w792, "EventStartupChecks"=T29 {"Timestamp"=1.0, "ILCVersionsOk"=TRUE, "DCAVersionsOk"=FALSE, "ILCFirmwareOk"=TRUE, "DCAFirmwareOk"=FALSE, "ILCStatusOk"=TRUE, "DCAStatusOk"=FALSE}, "M1M3SAL in"=w793) -> ("error out"=w791:errorcluster, "M1M3SAL out"=w790:refnum<class "M1M3SAL.lvclass">)  [unwired: 7 in]
      }
      event "StatusChecksGo": Value Change {
        n393 = event-data() -> ()  [unwired: 1 in, 6 out]
        n394 = call-dynamic "logStatusChecks.vi"("error in (no error)"=w797, "EventStatusChecks"=T30 {"Timestamp"=1.0, "ILCResetOk"=TRUE, "DCAResetOk"=FALSE, "ILCPowerOk"=TRUE, "DCAPowerOk"=FALSE}, "M1M3SAL in"=w798) -> ("error out"=w794:errorcluster, "M1M3SAL out"=w795:refnum<class "M1M3SAL.lvclass">)  [unwired: 7 in]
      }
      event "SummaryStateGo": Value Change {
        n395 = event-data() -> ()  [unwired: 1 in, 6 out]
        n396 = call-dynamic "logSummaryState.vi"("error in (no error)"=w799, "EventSummaryState"=T31 {"Timestamp"=1.0, "SummaryStates"=enum."DisabledState"}, "M1M3SAL in"=w803) -> ("error out"=w800:errorcluster, "M1M3SAL out"=w801:refnum<class "M1M3SAL.lvclass">)  [unwired: 7 in]
      }
      event "Stop": Value Change {
        n397 = event-data() -> ()  [unwired: 1 in, 3 out]
        n398 = local read "Stop"() -> (w806:bool)
      }
    }
  }
  n399 = call "generateInternalShutdown.vi"("error in (no error)"=w43, "ShutdownEvent"=T1 {"Shutdown"=TRUE}, "UserEvents in"=w24) -> ("error out"=w39:errorcluster, "UserEvents out"=w38:refnum<class "UserEvents.lvclass">)  [unwired: 7 in]
  n400 = call-dynamic "stopService.vi"("error in (no error)"=w39, "M1M3SAL in"=w40) -> ("error out"=w37:errorcluster)  [unwired: 8 in, 1 out]
  n401 = call "destroyUserEvents.vi"("error in (no error)"=w37, "UserEvents in"=w38) -> ()  [unwired: 8 in, 2 out]
  "Ready?" <- FALSE ("Ready?")
